vi "doStep.vi"(8 "error in (no error)":errorcluster, 10 "stepName":T1, 11 "Stand in":refnum<class "Stand.lvclass">) -> (0 "error out":errorcluster, 3 "Stand out":refnum<class "Stand.lvclass">)   [LabVIEW 2019, in "Stand.lvclass"]
uses:
  Stand.lvclass
  D:/GIT H4000/H4000/src/Device_class/Device.lvclass
  TypeDef/Step_Name.ctl
  Stand.lvclass/Stand.ctl
  Device_class/Device.lvclass/Device.ctl
  TypeDef/Direction.ctl
  FPGA/TypeDef/DO index.ctl
  FPGA/TypeDef/AI index.ctl
  AI_class/AI.lvclass/AI.ctl
  AnalogComparator_class/AnalogComparator.lvclass/AnalogComparator.ctl
  TypeDef/Active Motor.ctl
  TypeDef/Motor N.ctl
  f638fa31-f737-482a-bde8-81f5a2056bae.vi
  AnalogComparator_class/GetStatus.vi
  NeedleValve_class/NeedleValve.lvclass
  FPGA_API_class/FPGA API.lvclass
  MessageInterface_class/MessageInterface.lvclass
  Valve_2DO_2DI_class/Valve_2DO_2DI.lvclass
  Device_class/Device.lvclass
  PM_Group_class/PM_Group.lvclass
  AI_class/AI.lvclass
  ExpFitter/ExpFitter.lvclass
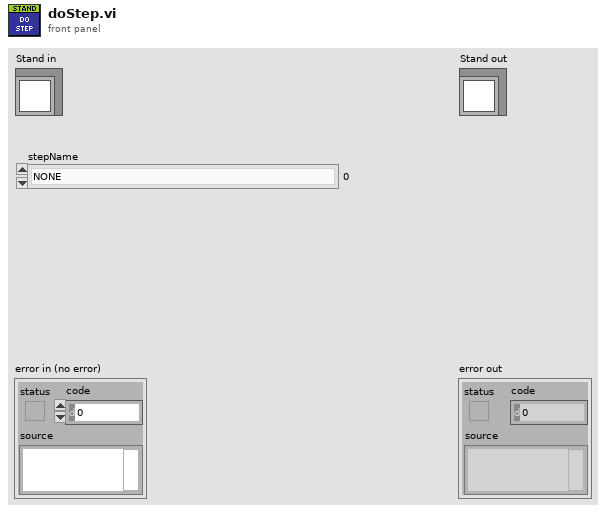
[diagram p1: front panel]
types:
  T1 = typedef "Step_Name.ctl" = enum16{"NONE", "Filling DUT", "Filling Chamber", "Pressure Up DUT", "Abrupt Pressure Release DUT", "Smooth Pressure Release DUT", "Pressure Up Chamber", "Abrupt Pressure Release Chamber", "Smooth Pressure Release Chamber", "Measuring leakage sensor 41.3", "Measuring leakage burette 42", "Low Pressure DUT", "Low Pressure Chamber", "Low Pressure HPP", "ALARM", "Open Air", "MicroStep DUT", "MicroStep CMBR", "Stop Pump"}
  T2 = typedef "Direction.ctl" = enum16{"None", "Chamber", "DUT"}
  T3 = typedef "Active Motor.ctl" = cluster{"Active":bool, "MotorN":T4}
  T4 = typedef "Motor N.ctl" = enum16{"M12", "M21", "M24"}
  T5 = typedef "DO index.ctl" = u8
  T6 = typedef "AI index.ctl" = u8
  T7 = typedef "AI_Data.ctl" = cluster{"Stat Data":T8, "OutOfRangeMax":bool, "OutOfRangeMin":bool, "HIHI":bool, "HI":bool, "LO":bool, "LOLO":bool}
  T8 = typedef "AI Statistics Data.ctl" = cluster{"raw mean":dbl, "scl mean":dbl, "raw mean 1Hz":dbl, "scl mean 1Hz":dbl, "raw standard deviation":dbl, "raw max value":dbl, "raw min value":dbl}
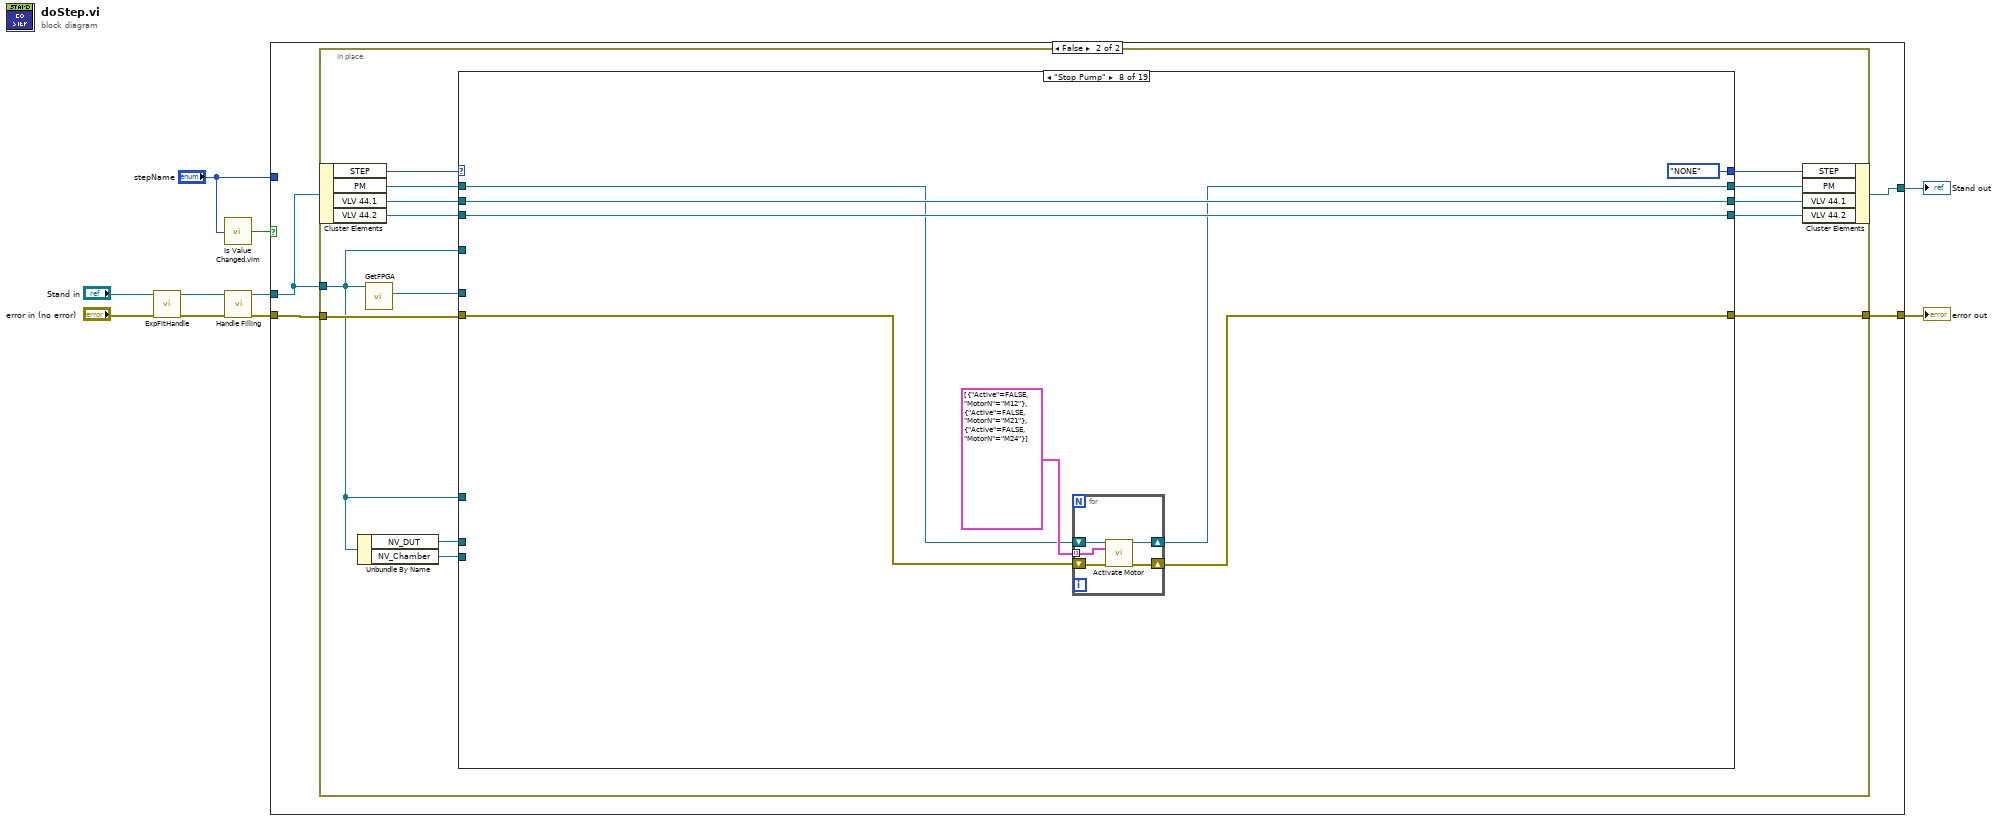
[diagram p0: block diagram]
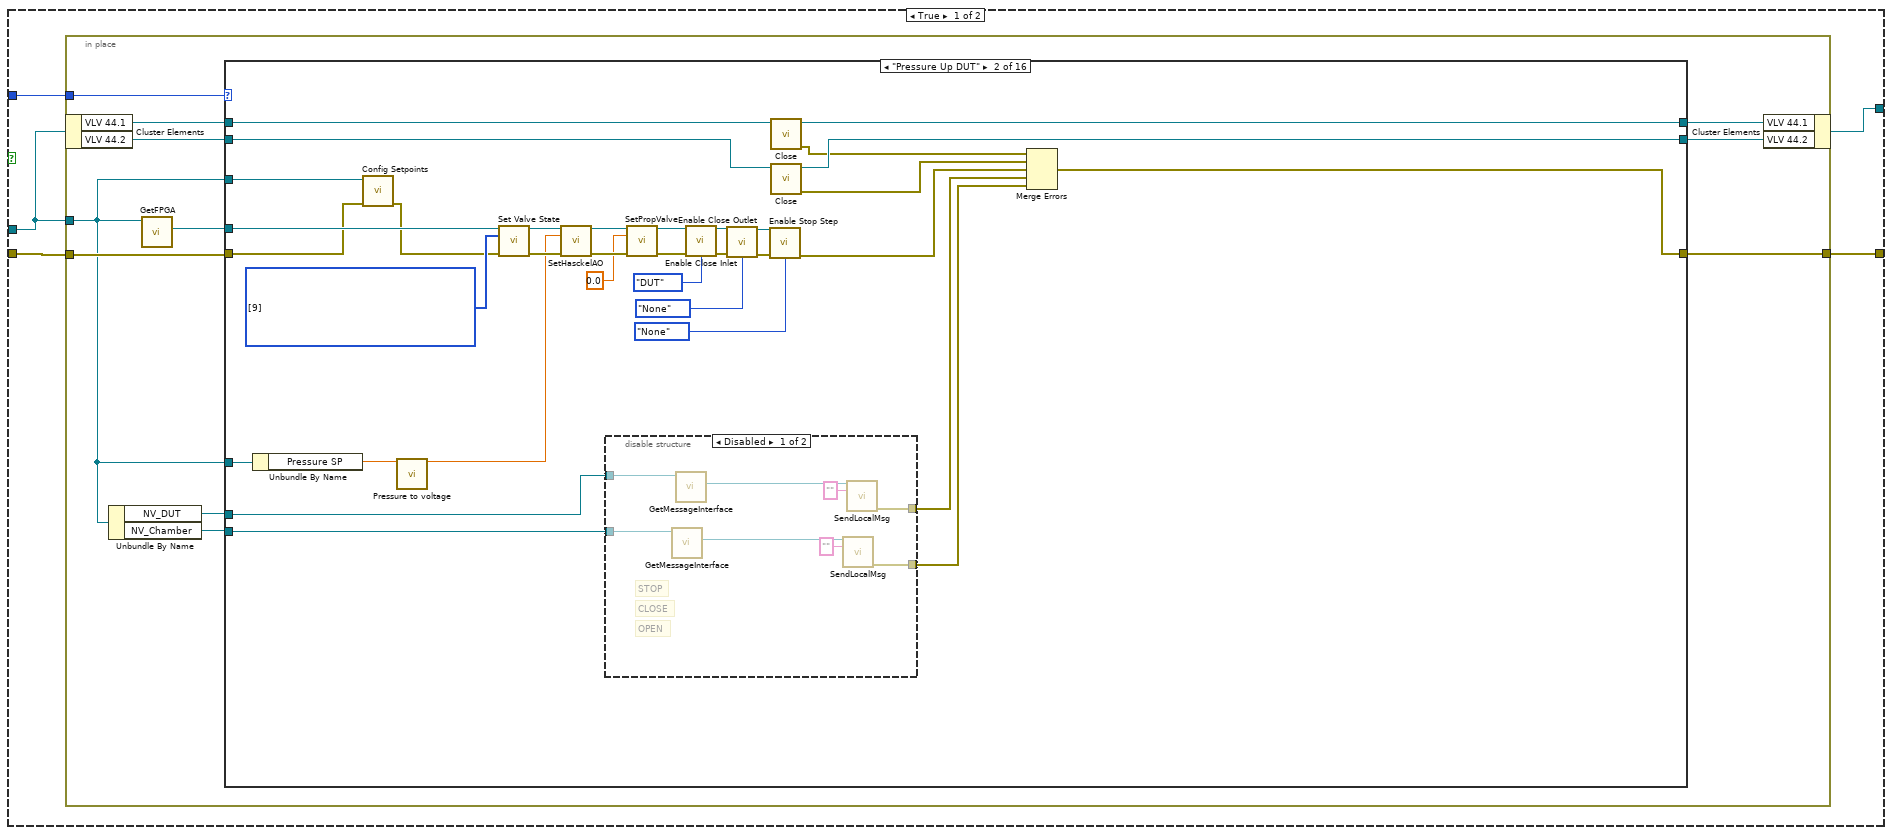
[diagram p2: hidden frame]
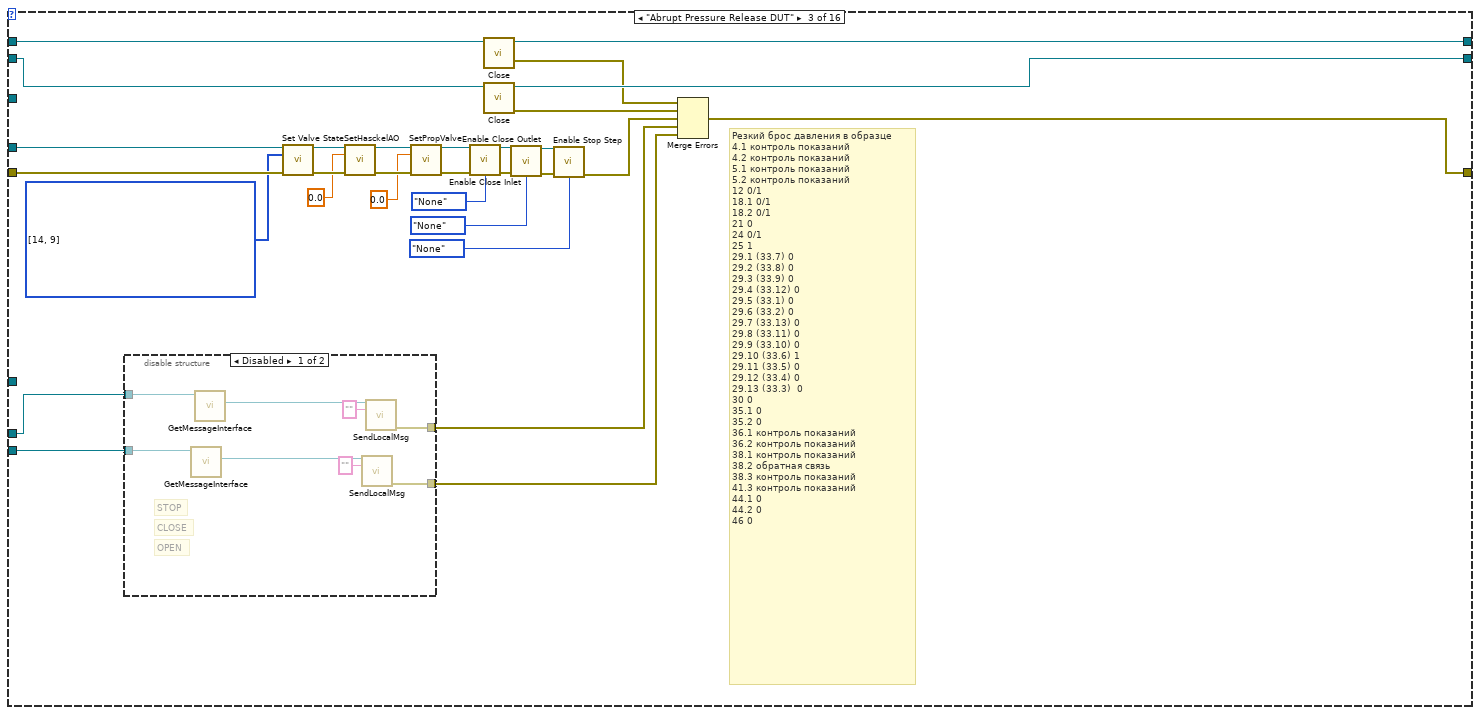
[diagram p5: hidden frame]
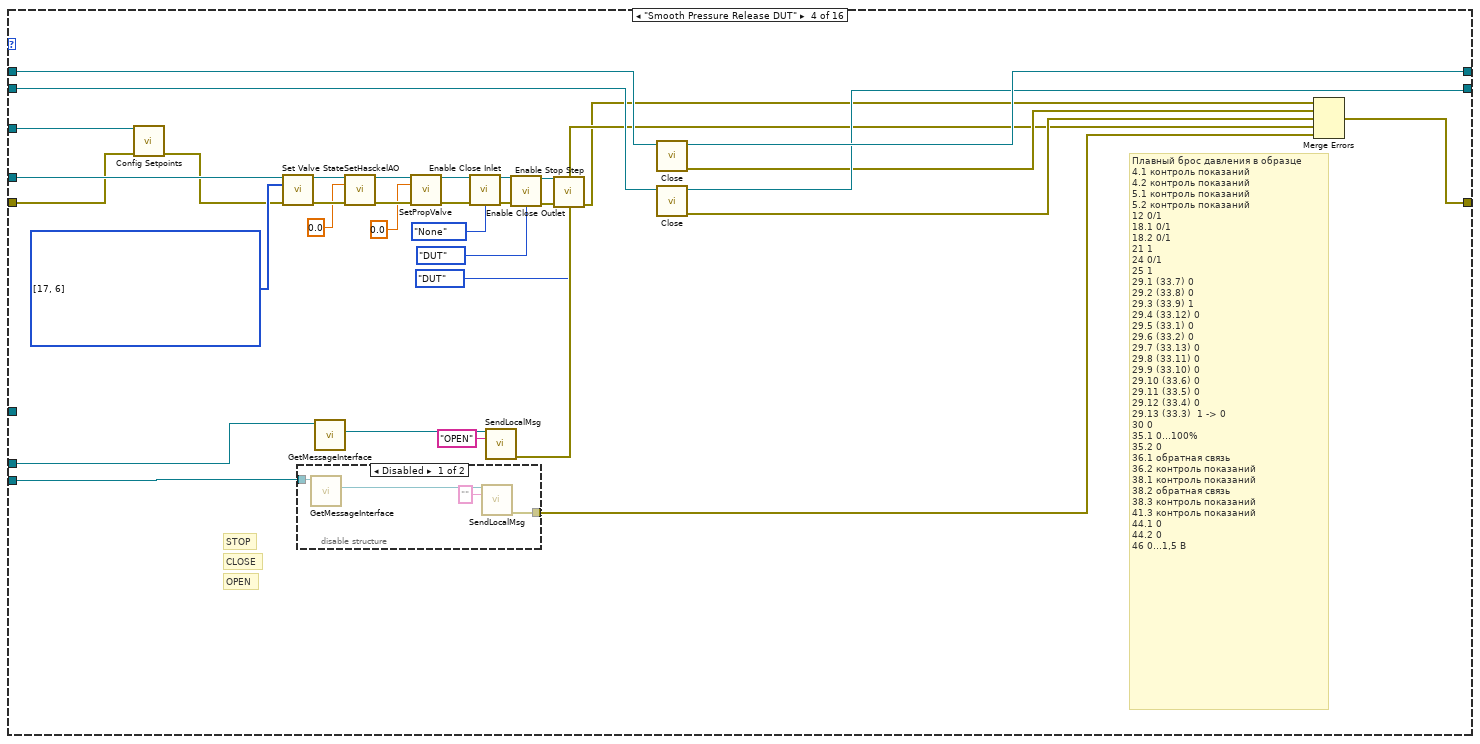
[diagram p7: hidden frame]
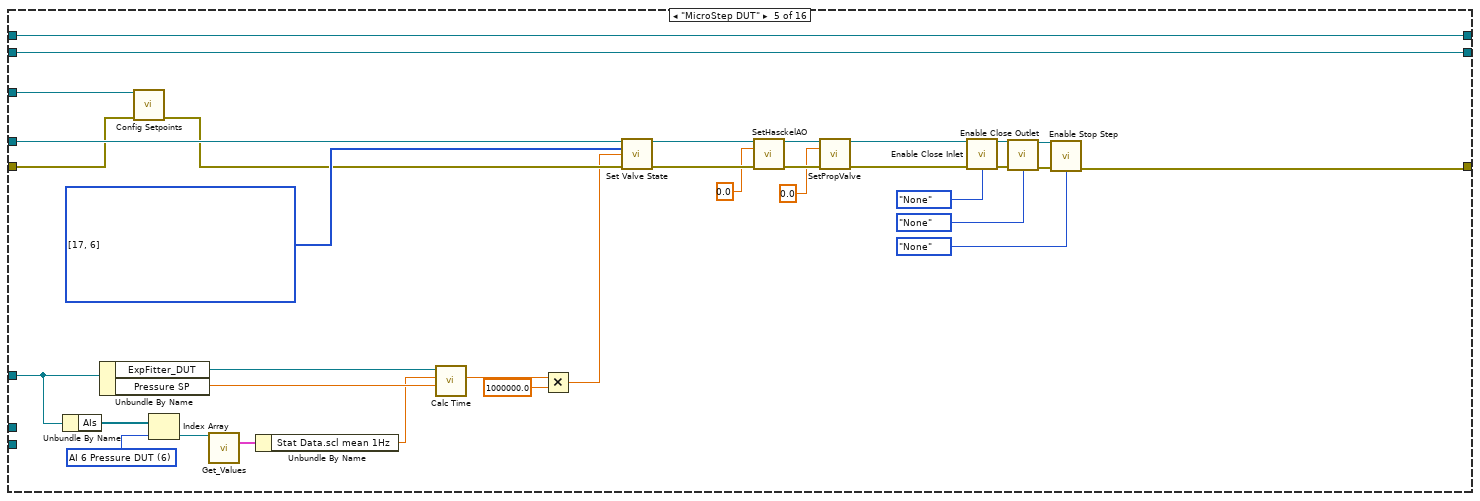
[diagram p9: hidden frame]
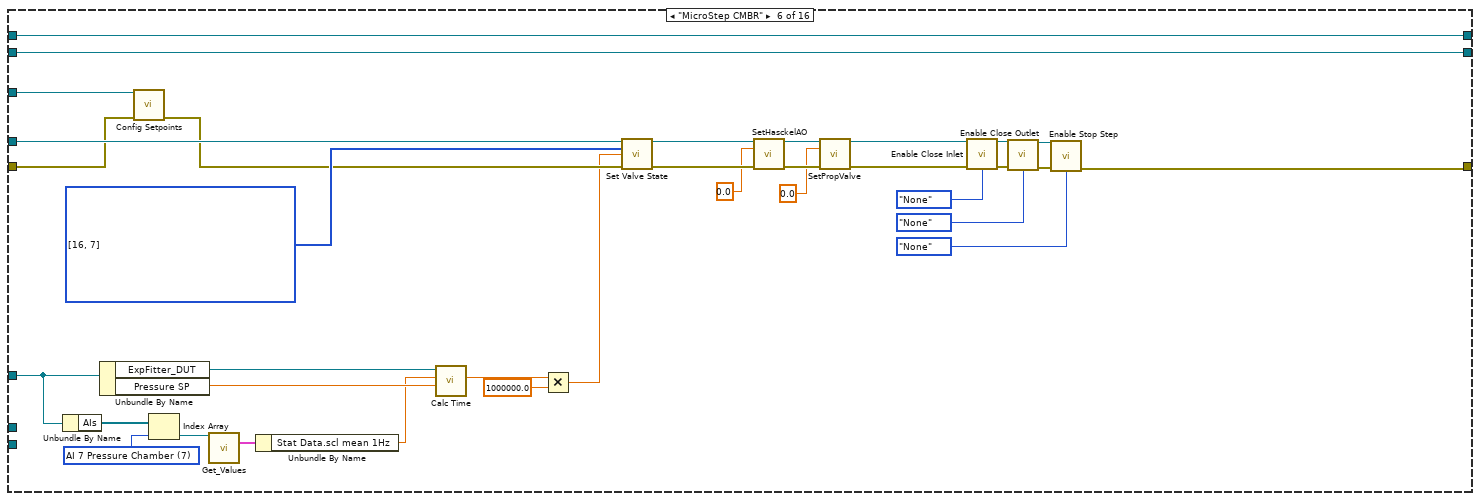
[diagram p10: hidden frame]
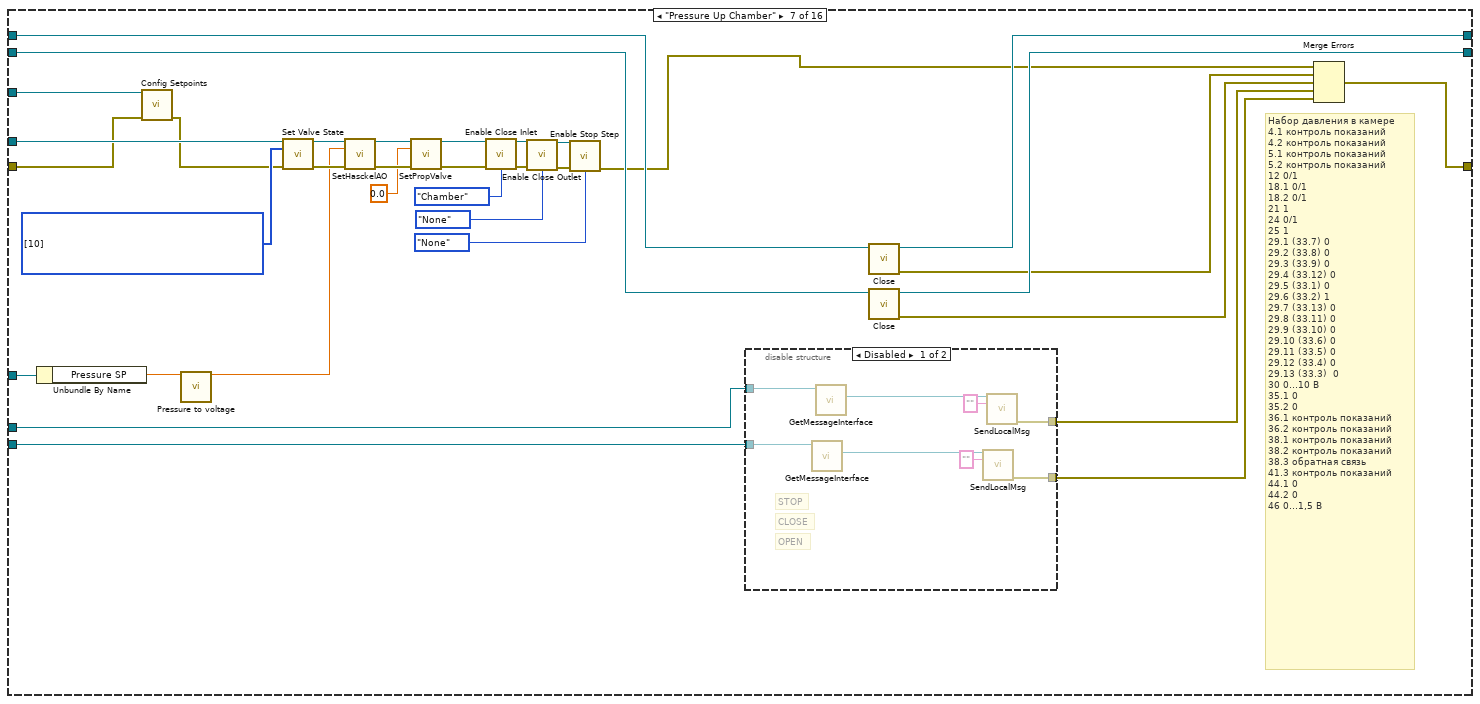
[diagram p11: hidden frame]
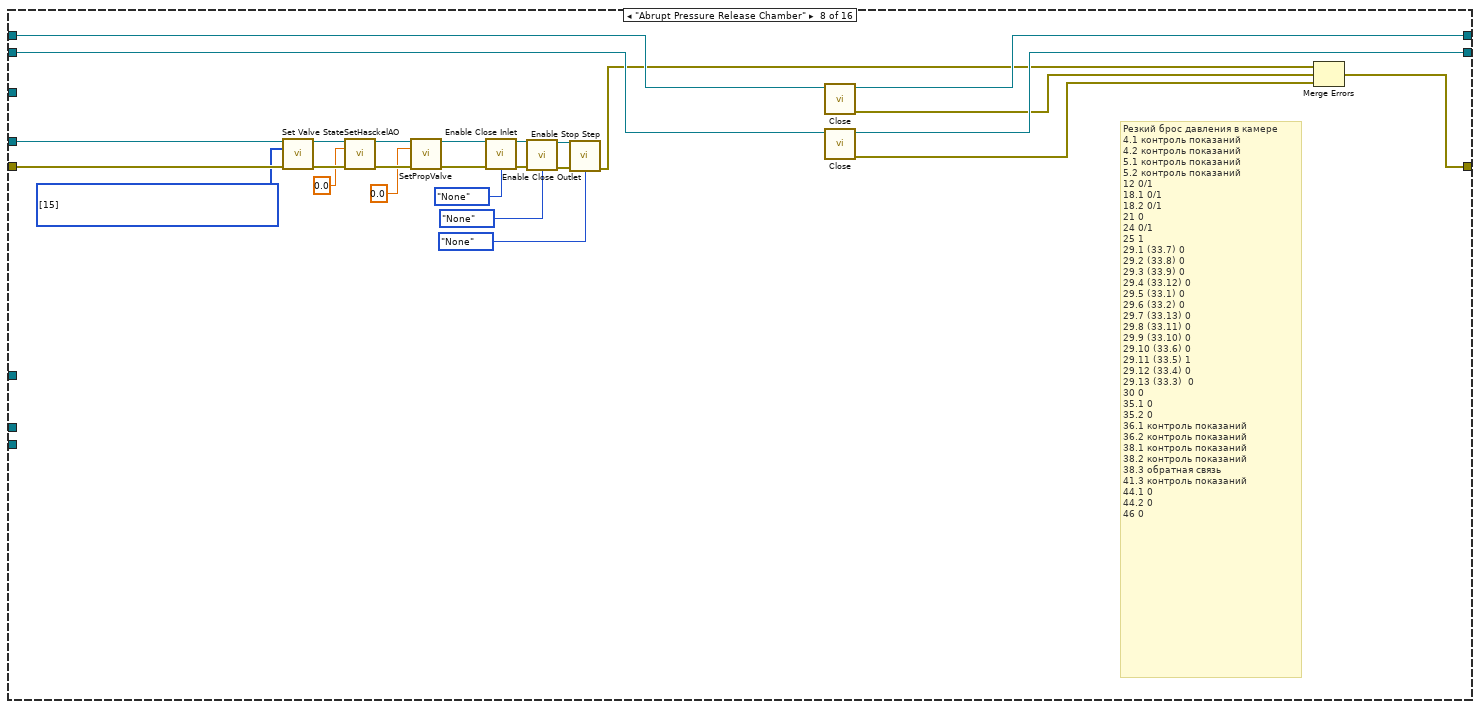
[diagram p13: hidden frame]
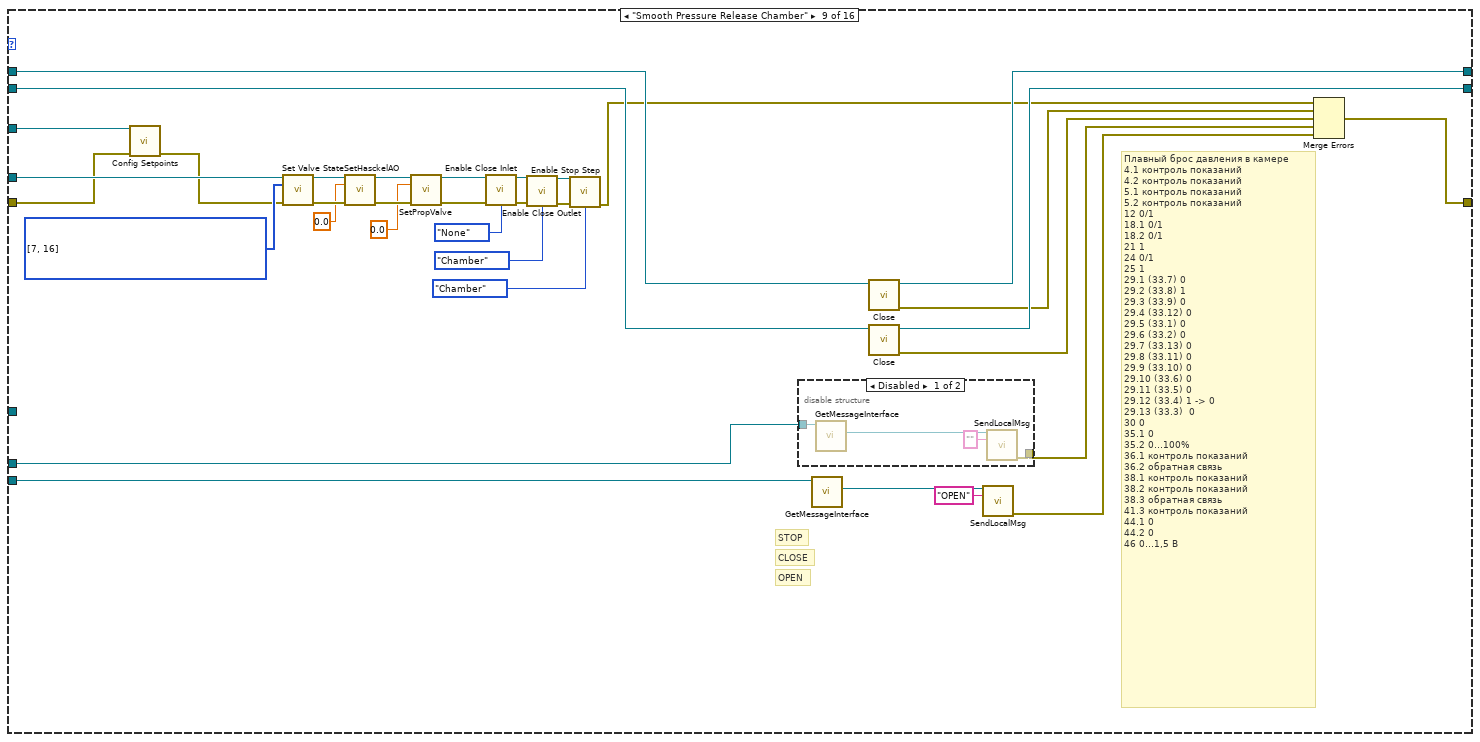
[diagram p14: hidden frame]
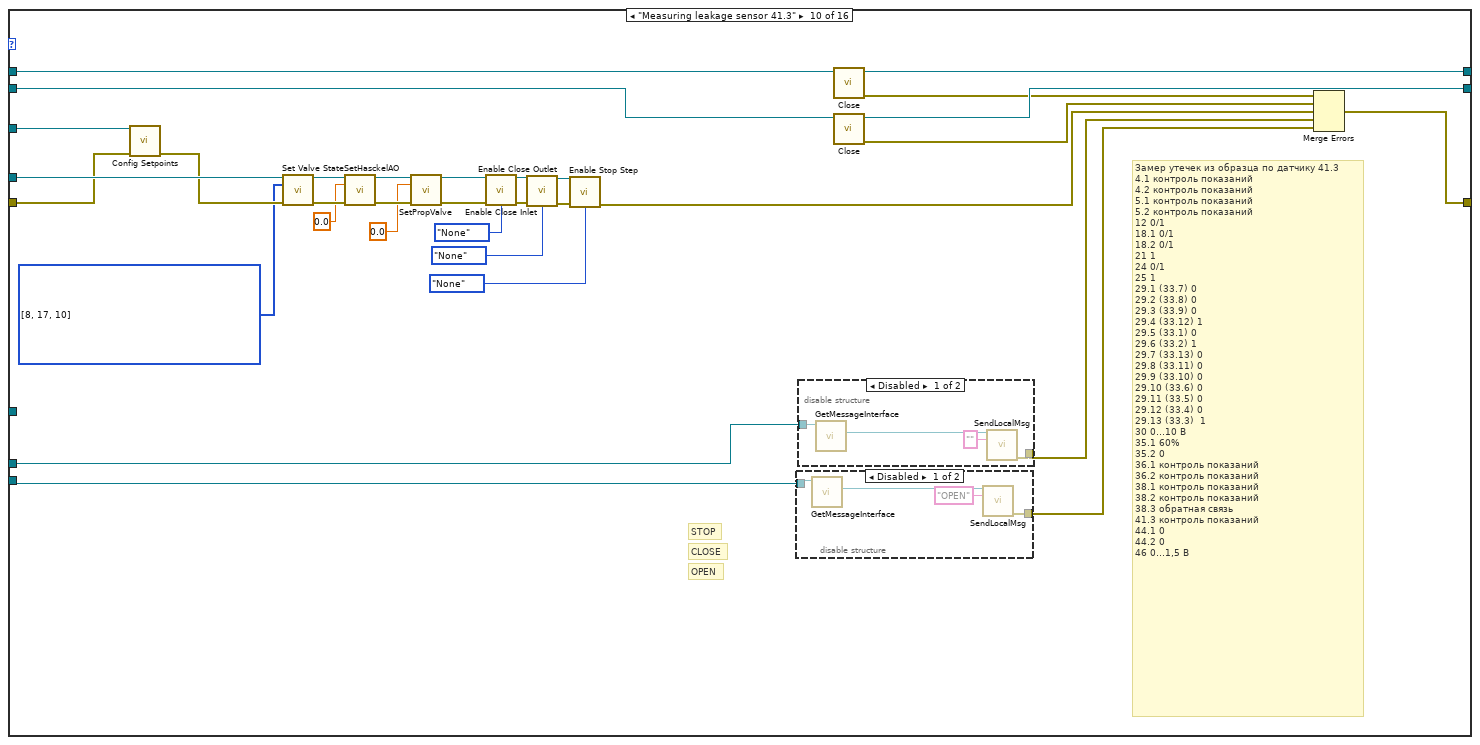
[diagram p16: hidden frame]
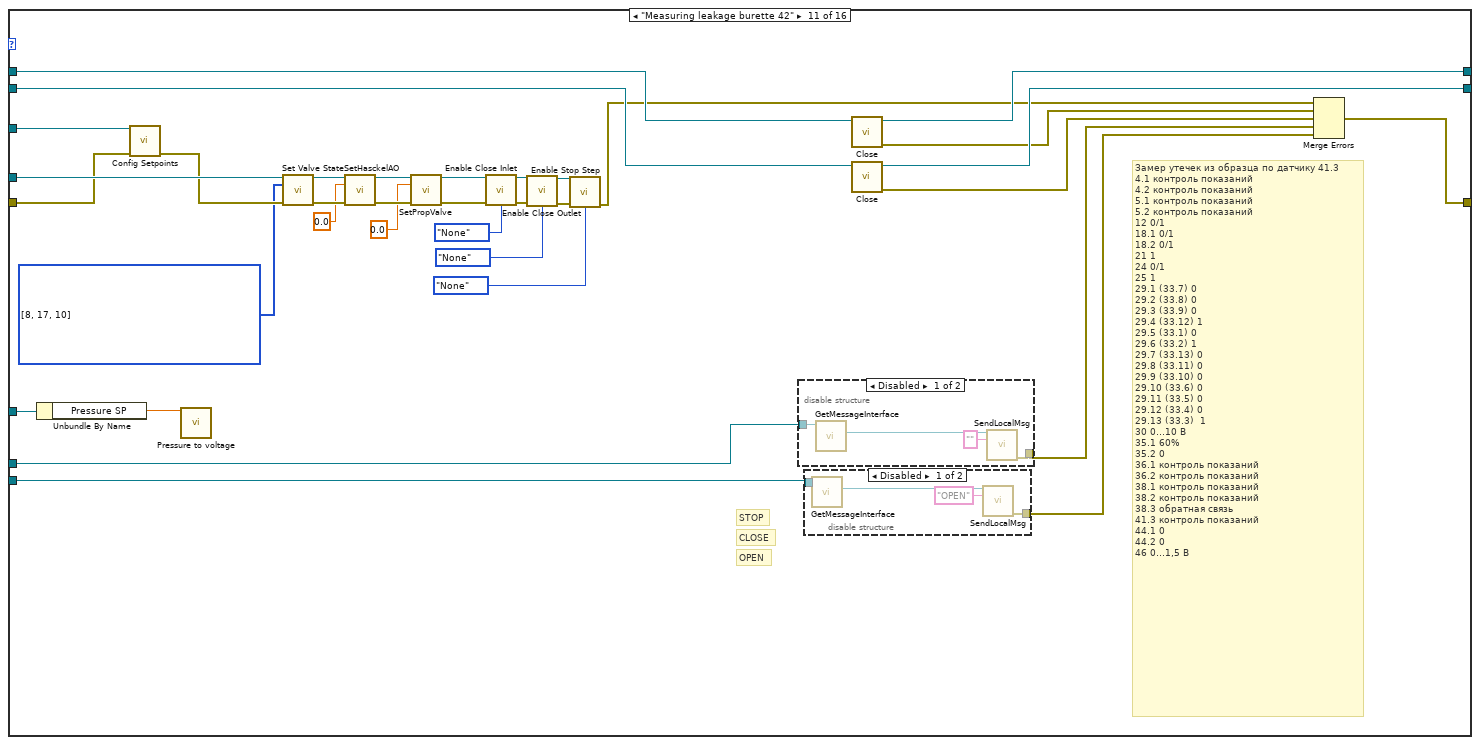
[diagram p19: hidden frame]
diagram:
  n1 = call "ExpFitHandle.vi"("error in (no error)"="error in (no error)", "Stand in"="Stand in") -> ("error out"=w3:errorcluster, "Stand out"=w4:refnum<class "Stand.lvclass">)  [unwired: 8 in]
  n2 = call "Is Value Changed.vim"("value"="stepName") -> ("changed or first call?"=w9:bool)
  n3 = call "Handle Filling.vi"("error in (no error)"=w3, "Stand in"=w4) -> ("error out"=w2:errorcluster, "Stand out"=w1:refnum<class "Stand.lvclass">)  [unwired: 8 in]
  n4 = case shown="False" w9 {
    tunnel: "stepName" -> [w15 _]
    tunnel: w1 -> [w13 w582]
    tunnel: w2 -> [w14 w583]
    tunnel: [w12 w581] -> w8
    tunnel: [w11 w580] -> w7
    frame True {
      n5 = in-place {
        in-place-border: w15 -> [w26]
        in-place-border: [w25] -> w11
        in-place-border: w14 -> [w24]
        in-place-border: w13 -> [w16]
        n6 = in-place-cluster #1(w13) -> ("VLV 44.1"=w22:refnum<class "Valve_2DO_2DI.lvclass">, "VLV 44.2"=w21:refnum<class "Valve_2DO_2DI.lvclass">)
        n7 = Unbundle By Name(w16) -> ("NV_DUT"=w18:refnum<class "NeedleValve.lvclass">, "NV_Chamber"=w17:refnum<class "NeedleValve.lvclass">)
        n8 = call "GetFPGA.vi"("Device in"=w16) -> ("FPGA API.lvclass"=w23:refnum<class "FPGA API.lvclass">)  [unwired: 10 in]
        n9 = case shown="\"Pressure Up DUT\"" w26 {
          tunnel: w24 -> [w29 w34 w101 w113 w160 w194 w217 w283 w285 w325 w364 w433 w471 w509 w543 w548]
          tunnel: [w29 w53 w91 w134 w166 w200 w239 w273 w308 w344 w385 w423 w461 w499 w533 w567] -> w25
          tunnel: w22 -> [w28 w58 w95 w138 w176 w210 w244 w277 w312 w348 w390 w427 w465 w503 w537 w569]
          tunnel: w21 -> [w27 w55 w93 w136 w175 w209 w241 w275 w310 w346 w387 w425 w463 w501 w535 w568]
          tunnel: w23 -> [_ w59 w96 w139 w177 w211 w245 w278 w313 w349 w391 w428 w466 w504 w538 w549]
          tunnel: w16 -> [_ w57 _ _ w153 w187 w243 _ _ _ w389 _ _ _ _ _]
          tunnel: [w28 w56 w94 w137 w176 w210 w242 w276 w311 w347 w388 w426 w464 w502 w536 w569] -> w20
          tunnel: [w27 w54 w92 w135 w175 w209 w240 w274 w309 w345 w386 w424 w462 w500 w534 w568] -> w19
          tunnel: w18 -> [_ w52 w90 w131 _ _ w236 _ w305 w341 w382 w420 w458 w496 _ w566]
          tunnel: w17 -> [_ w50 w88 w129 _ _ w234 _ w303 w339 w380 w418 w456 w494 _ w564]
          tunnel: w16 -> [_ w35 _ w114 w161 w195 w218 _ w286 w326 w365 _ _ _ _ _]
          frame "NONE", Default {
          }
          frame "Pressure Up DUT" {
            w39 = T5[] [9] items=["DO 0 [KP1] [M12]", "DO 1 [ON KP2] [M21]", "DO 2 [ON KP3] [M24]", "DO 3 [WATER Y18.1 [DO3]]", "DO 4 [WATER Y18.2 [DO4]]", "DO 5 [KP6 Y29.1 33.7]", "DO 6 [KP7 Y29.2 33.8]", "DO 7 [KP8 Y29.3 33.9]", "DO 8 [KP9 Y29.4  33.12]", "DO 9 [KP10 Y29.5 33.1]", "DO 10 [KP11 Y29.6 33.2]", "DO 11 [KP12 Y29.7  33.13]", "DO 12 [KP13 Y29.8  33.11]", "DO 13 [KP14 Y29.9 33.10]", "DO 14 [KP15 Y29.10  33.6]", "DO 15 [KP16 Y29.11  33.5]", "DO 16 [KP17 Y29.12  33.4]", "DO 17 [KP18 Y29.13 33.3]", "DO 18 [AIR KP19]", "DO 19 [STEP DRIVE EN KP20]", "DO 20 [KP21 Y44.1 OPEN]", "DO 21 [ KP22 Y44.1 CLOSE]", "DO 22 [ KP23 Y44.2 OPEN]", "DO 23", "DO 24 [STEP DRIVE 1]", "DO 25 [STEP DRIVE 2]"] ("#DO")
            n10 = Unbundle By Name(w57) -> ("Pressure SP"=w37:dbl)
            n11 = call "Config Setpoints.vi"("reference in"=w35, "error in (no error)"=w34) -> ("error out"=w33:errorcluster)  [unwired: 13 in]
            n12 = call "Pressure to voltage.vi"("Pressure SP"=w37) -> ("Voltage"=w36:dbl)  [unwired: 14 in]
            n13 = call "Set Valve State.vi"("reference in"=w59, "#DO"=w39, "error in (no error)"=w33) -> ("reference out"=w63:refnum<class "FPGA API.lvclass">, "error out"=w62:errorcluster)  [unwired: 11 in]
            n14 = call-dynamic "SetHasckelAO.vi"("FPGA API in"=w63, "Haskel in"=w36, "error in (no error)"=w62) -> ("FPGA API out"=w61:refnum<class "FPGA API.lvclass">, "error out"=w60:errorcluster)  [unwired: 11 in]
            n15 = disable-structure shown="Disabled" {
              disable-tunnel: w52 -> [w71 _]
              disable-tunnel: [w69 _] -> w51
              disable-tunnel: w50 -> [w67 _]
              disable-tunnel: [w64 _] -> w40
              frame Disabled {
                # "OPEN"
                # "CLOSE"
                # "STOP"
                n16 = call "GetMessageInterface.vi"("Device in"=w67) -> ("MessageInterface"=w68:refnum<class "MessageInterface.lvclass">)  [unwired: 10 in]
                n17 = call "GetMessageInterface.vi"("Device in"=w71) -> ("MessageInterface"=w70:refnum<class "MessageInterface.lvclass">)  [unwired: 10 in]
                n18 = call-dynamic "SendLocalMsg.vi"("reference in"=w68, "name"="") -> ("error out"=w64:errorcluster)  [unwired: 11 in, 2 out]
                n19 = call-dynamic "SendLocalMsg.vi"("reference in"=w70, "name"="") -> ("error out"=w69:errorcluster)  [unwired: 11 in, 2 out]
              }
              frame Enabled {
              }
            }
            n20 = call-dynamic "SetPropValve.vi"("FPGA API in"=w61, "AO 1"=0.0, "error in (no error)"=w60) -> ("FPGA API out"=w49:refnum<class "FPGA API.lvclass">, "error out"=w48:errorcluster)  [unwired: 11 in]
            n21 = call-dynamic "Enable Close Inlet.vi"("FPGA API in"=w49, "error in (no error)"=w48, "Direction"=Direction."DUT") -> ("FPGA API out"=w46:refnum<class "FPGA API.lvclass">, "error out"=w45:errorcluster)  [unwired: 11 in]
            n22 = call-dynamic "Enable Close Outlet.vi"("FPGA API in"=w46, "error in (no error)"=w45, "Direction"=Direction."None") -> ("FPGA API out"=w43:refnum<class "FPGA API.lvclass">, "error out"=w42:errorcluster)  [unwired: 11 in]
            n23 = call-dynamic "Enable Stop Step.vi"("FPGA API in"=w43, "error in (no error)"=w42, "Direction"=Direction."None") -> ("error out"=w32:errorcluster)  [unwired: 11 in, 1 out]
            n24 = call "Close.vi"("Pump_1AI_1DO_2DI in"=w58) -> ("error out"=w30:errorcluster, "Pump_1AI_1DO_2DI out"=w56:refnum<class "Valve_2DO_2DI.lvclass">)  [unwired: 9 in]
            n25 = call "Close.vi"("Pump_1AI_1DO_2DI in"=w55) -> ("error out"=w31:errorcluster, "Pump_1AI_1DO_2DI out"=w54:refnum<class "Valve_2DO_2DI.lvclass">)  [unwired: 9 in]
            n26 = Merge Errors(w30, w31, w32, w51, w40) -> (w53:errorcluster)
          }
          frame "Abrupt Pressure Release DUT" {
            w76 = T5[] [14, 9] items=["DO 0 [KP1] [M12]", "DO 1 [ON KP2] [M21]", "DO 2 [ON KP3] [M24]", "DO 3 [WATER Y18.1 [DO3]]", "DO 4 [WATER Y18.2 [DO4]]", "DO 5 [KP6 Y29.1 33.7]", "DO 6 [KP7 Y29.2 33.8]", "DO 7 [KP8 Y29.3 33.9]", "DO 8 [KP9 Y29.4  33.12]", "DO 9 [KP10 Y29.5 33.1]", "DO 10 [KP11 Y29.6 33.2]", "DO 11 [KP12 Y29.7  33.13]", "DO 12 [KP13 Y29.8  33.11]", "DO 13 [KP14 Y29.9 33.10]", "DO 14 [KP15 Y29.10  33.6]", "DO 15 [KP16 Y29.11  33.5]", "DO 16 [KP17 Y29.12  33.4]", "DO 17 [KP18 Y29.13 33.3]", "DO 18 [AIR KP19]", "DO 19 [STEP DRIVE EN KP20]", "DO 20 [KP21 Y44.1 OPEN]", "DO 21 [ KP22 Y44.1 CLOSE]", "DO 22 [ KP23 Y44.2 OPEN]", "DO 23", "DO 24 [STEP DRIVE 1]", "DO 25 [STEP DRIVE 2]"] ("#DO")
            # "Резкий брос давления в образце\n4.1\tконтроль показаний\n4.2\tконтроль показаний\n5.1\tконтроль показаний\n5.2\tконтроль показаний\n12\t0/1\n18.1\t0/1\n18.2\t0/1\n21\t0\n24\t0/1\n25\t1\n29.1 (33.7)\t0\n29.2 (33.8)\t0\n29.3 (33.9)\t0\n29.4 (33.12)\t0\n29.5 (33.1)\t0\n29.6 (33.2)\t0\n29.7 (33.13)\t0\n29.8 (33.11)\t0\n29.9 (33.10)\t0\n29.10 (33.6)\t1\n29.11 (33.5)\t0\n29.12 (33.4)\t0\n29.13 (33.3) \t0\n30\t0\n35.1\t0\n35.2\t0\n36.1\tконтроль показаний\n36.2\tконтроль показаний\n38.1\tконтроль показаний\n38.2\tобратная связь\n38.3\tконтроль показаний\n41.3\tконтроль показаний\n44.1\t0\n44.2\t0\n46\t0"
            n27 = disable-structure shown="Disabled" {
              disable-tunnel: w90 -> [w109 _]
              disable-tunnel: [w107 _] -> w89
              disable-tunnel: w88 -> [w105 _]
              disable-tunnel: [w102 _] -> w78
              frame Disabled {
                # "OPEN"
                # "CLOSE"
                # "STOP"
                n28 = call "GetMessageInterface.vi"("Device in"=w105) -> ("MessageInterface"=w106:refnum<class "MessageInterface.lvclass">)  [unwired: 10 in]
                n29 = call "GetMessageInterface.vi"("Device in"=w109) -> ("MessageInterface"=w108:refnum<class "MessageInterface.lvclass">)  [unwired: 10 in]
                n30 = call-dynamic "SendLocalMsg.vi"("reference in"=w106, "name"="") -> ("error out"=w102:errorcluster)  [unwired: 11 in, 2 out]
                n31 = call-dynamic "SendLocalMsg.vi"("reference in"=w108, "name"="") -> ("error out"=w107:errorcluster)  [unwired: 11 in, 2 out]
              }
              frame Enabled {
              }
            }
            n32 = call "Set Valve State.vi"("reference in"=w96, "#DO"=w76, "error in (no error)"=w101) -> ("reference out"=w100:refnum<class "FPGA API.lvclass">, "error out"=w99:errorcluster)  [unwired: 11 in]
            n33 = call-dynamic "SetHasckelAO.vi"("FPGA API in"=w100, "Haskel in"=0.0, "error in (no error)"=w99) -> ("FPGA API out"=w98:refnum<class "FPGA API.lvclass">, "error out"=w97:errorcluster)  [unwired: 11 in]
            n34 = call-dynamic "SetPropValve.vi"("FPGA API in"=w98, "AO 1"=0.0, "error in (no error)"=w97) -> ("FPGA API out"=w87:refnum<class "FPGA API.lvclass">, "error out"=w86:errorcluster)  [unwired: 11 in]
            n35 = call-dynamic "Enable Close Inlet.vi"("FPGA API in"=w87, "error in (no error)"=w86, "Direction"=Direction."None") -> ("FPGA API out"=w84:refnum<class "FPGA API.lvclass">, "error out"=w83:errorcluster)  [unwired: 11 in]
            n36 = call "Close.vi"("Pump_1AI_1DO_2DI in"=w95) -> ("error out"=w73:errorcluster, "Pump_1AI_1DO_2DI out"=w94:refnum<class "Valve_2DO_2DI.lvclass">)  [unwired: 9 in]
            n37 = call "Close.vi"("Pump_1AI_1DO_2DI in"=w93) -> ("error out"=w74:errorcluster, "Pump_1AI_1DO_2DI out"=w92:refnum<class "Valve_2DO_2DI.lvclass">)  [unwired: 9 in]
            n38 = call-dynamic "Enable Close Outlet.vi"("FPGA API in"=w84, "error in (no error)"=w83, "Direction"=Direction."None") -> ("FPGA API out"=w81:refnum<class "FPGA API.lvclass">, "error out"=w80:errorcluster)  [unwired: 11 in]
            n39 = call-dynamic "Enable Stop Step.vi"("FPGA API in"=w81, "error in (no error)"=w80, "Direction"=Direction."None") -> ("error out"=w72:errorcluster)  [unwired: 11 in, 1 out]
            n40 = Merge Errors(w73, w74, w72, w89, w78) -> (w91:errorcluster)
          }
          frame "Smooth Pressure Release DUT" {
            w116 = T5[] [17, 6] items=["DO 0 [KP1] [M12]", "DO 1 [ON KP2] [M21]", "DO 2 [ON KP3] [M24]", "DO 3 [WATER Y18.1 [DO3]]", "DO 4 [WATER Y18.2 [DO4]]", "DO 5 [KP6 Y29.1 33.7]", "DO 6 [KP7 Y29.2 33.8]", "DO 7 [KP8 Y29.3 33.9]", "DO 8 [KP9 Y29.4  33.12]", "DO 9 [KP10 Y29.5 33.1]", "DO 10 [KP11 Y29.6 33.2]", "DO 11 [KP12 Y29.7  33.13]", "DO 12 [KP13 Y29.8  33.11]", "DO 13 [KP14 Y29.9 33.10]", "DO 14 [KP15 Y29.10  33.6]", "DO 15 [KP16 Y29.11  33.5]", "DO 16 [KP17 Y29.12  33.4]", "DO 17 [KP18 Y29.13 33.3]", "DO 18 [AIR KP19]", "DO 19 [STEP DRIVE EN KP20]", "DO 20 [KP21 Y44.1 OPEN]", "DO 21 [ KP22 Y44.1 CLOSE]", "DO 22 [ KP23 Y44.2 OPEN]", "DO 23", "DO 24 [STEP DRIVE 1]", "DO 25 [STEP DRIVE 2]"] ("#DO")
            # "OPEN"
            # "CLOSE"
            # "STOP"
            # "Плавный брос давления в образце\n4.1\tконтроль показаний\n4.2\tконтроль показаний\n5.1\tконтроль показаний\n5.2\tконтроль показаний\n12\t0/1\n18.1\t0/1\n18.2\t0/1\n21\t1\n24\t0/1\n25\t1\n29.1 (33.7)\t0\n29.2 (33.8)\t0\n29.3 (33.9)\t1\n29.4 (33.12)\t0\n29.5 (33.1)\t0\n29.6 (33.2)\t0\n29.7 (33.13)\t0\n29.8 (33.11)\t0\n29.9 (33.10)\t0\n29.10 (33.6)\t0\n29.11 (33.5)\t0\n29.12 (33.4)\t0\n29.13 (33.3) \t1 -> 0\n30\t0\n35.1\t0…100%\n35.2\t0\n36.1\tобратная связь\n36.2\tконтроль показаний\n38.1\tконтроль показаний\n38.2\tобратная связь\n38.3\tконтроль показаний\n41.3\tконтроль показаний\n44.1\t0\n44.2\t0\n46\t0…1,5 В"
            n41 = call "Config Setpoints.vi"("reference in"=w114, "error in (no error)"=w113) -> ("error out"=w112:errorcluster)  [unwired: 13 in]
            n42 = call "Set Valve State.vi"("reference in"=w139, "#DO"=w116, "error in (no error)"=w112) -> ("reference out"=w143:refnum<class "FPGA API.lvclass">, "error out"=w142:errorcluster)  [unwired: 11 in]
            n43 = disable-structure shown="Disabled" {
              disable-tunnel: w129 -> [w147 _]
              disable-tunnel: [w146 _] -> w118
              frame Disabled {
                n44 = call "GetMessageInterface.vi"("Device in"=w147) -> ("MessageInterface"=w145:refnum<class "MessageInterface.lvclass">)  [unwired: 10 in]
                n45 = call-dynamic "SendLocalMsg.vi"("reference in"=w145, "name"="") -> ("error out"=w146:errorcluster)  [unwired: 11 in, 2 out]
              }
              frame Enabled {
              }
            }
            n46 = call "GetMessageInterface.vi"("Device in"=w131) -> ("MessageInterface"=w111:refnum<class "MessageInterface.lvclass">)  [unwired: 10 in]
            n47 = call-dynamic "SetHasckelAO.vi"("FPGA API in"=w143, "Haskel in"=0.0, "error in (no error)"=w142) -> ("FPGA API out"=w141:refnum<class "FPGA API.lvclass">, "error out"=w140:errorcluster)  [unwired: 11 in]
            n48 = call-dynamic "SetPropValve.vi"("FPGA API in"=w141, "AO 1"=0.0, "error in (no error)"=w140) -> ("FPGA API out"=w128:refnum<class "FPGA API.lvclass">, "error out"=w127:errorcluster)  [unwired: 11 in]
            n49 = call-dynamic "Enable Close Inlet.vi"("FPGA API in"=w128, "error in (no error)"=w127, "Direction"=Direction."None") -> ("FPGA API out"=w125:refnum<class "FPGA API.lvclass">, "error out"=w124:errorcluster)  [unwired: 11 in]
            n50 = call-dynamic "SendLocalMsg.vi"("reference in"=w111, "name"="OPEN") -> ("error out"=w130:errorcluster)  [unwired: 11 in, 2 out]
            n51 = call-dynamic "Enable Close Outlet.vi"("FPGA API in"=w125, "error in (no error)"=w124, "Direction"=Direction."DUT") -> ("FPGA API out"=w122:refnum<class "FPGA API.lvclass">, "error out"=w121:errorcluster)  [unwired: 11 in]
            n52 = call-dynamic "Enable Stop Step.vi"("FPGA API in"=w122, "error in (no error)"=w121, "Direction"=Direction."DUT") -> ("error out"=w120:errorcluster)  [unwired: 11 in, 1 out]
            n53 = call "Close.vi"("Pump_1AI_1DO_2DI in"=w138) -> ("error out"=w132:errorcluster, "Pump_1AI_1DO_2DI out"=w137:refnum<class "Valve_2DO_2DI.lvclass">)  [unwired: 9 in]
            n54 = call "Close.vi"("Pump_1AI_1DO_2DI in"=w136) -> ("error out"=w133:errorcluster, "Pump_1AI_1DO_2DI out"=w135:refnum<class "Valve_2DO_2DI.lvclass">)  [unwired: 9 in]
            n55 = Merge Errors(w120, w132, w133, w130, w118) -> (w134:errorcluster)
          }
          frame "MicroStep DUT" {
            w155 = T6 6 items=["AI 0 Cooling Station Level", "AI 1 Cooling Station Temp", "AI 2 Oil Supply Level", "AI 3 Oil Supply Temp", "AI 4 ", "AI 5 Pressure Haskel", "AI 6 Pressure DUT", "AI 7 Pressure Chamber", "AI 8 Pressure Air inlet", "AI 9 Pressure Air outlet", "AI 10 Pressure Messure Line"] ("AI index")
            w163 = T5[] [17, 6] items=["DO 0 [KP1] [M12]", "DO 1 [ON KP2] [M21]", "DO 2 [ON KP3] [M24]", "DO 3 [WATER Y18.1 [DO3]]", "DO 4 [WATER Y18.2 [DO4]]", "DO 5 [KP6 Y29.1 33.7]", "DO 6 [KP7 Y29.2 33.8]", "DO 7 [KP8 Y29.3 33.9]", "DO 8 [KP9 Y29.4  33.12]", "DO 9 [KP10 Y29.5 33.1]", "DO 10 [KP11 Y29.6 33.2]", "DO 11 [KP12 Y29.7  33.13]", "DO 12 [KP13 Y29.8  33.11]", "DO 13 [KP14 Y29.9 33.10]", "DO 14 [KP15 Y29.10  33.6]", "DO 15 [KP16 Y29.11  33.5]", "DO 16 [KP17 Y29.12  33.4]", "DO 17 [KP18 Y29.13 33.3]", "DO 18 [AIR KP19]", "DO 19 [STEP DRIVE EN KP20]", "DO 20 [KP21 Y44.1 OPEN]", "DO 21 [ KP22 Y44.1 CLOSE]", "DO 22 [ KP23 Y44.2 OPEN]", "DO 23", "DO 24 [STEP DRIVE 1]", "DO 25 [STEP DRIVE 2]"] ("#DO")
            n56 = Unbundle By Name(w153) -> ("AIs"=w154:refnum<class "AI.lvclass">[])
            n57 = Unbundle By Name(w153) -> ("ExpFitter_DUT"=w158:refnum<class "ExpFitter.lvclass">, "Pressure SP"=w152:dbl)
            n58 = call "Config Setpoints.vi"("reference in"=w161, "error in (no error)"=w160) -> ("error out"=w159:errorcluster)  [unwired: 13 in]
            n59 = Index Array(array=w154, index=w155) -> (element=w156:refnum<class "AI.lvclass">)
            n60 = call "Get_Values.vi"("reference in"=w156) -> ("Data"=w157:T7)  [unwired: 14 in]
            n61 = Unbundle By Name(w157) -> ("Stat Data.scl mean 1Hz"=w151:dbl)
            n62 = call "Calc Time.vi"("SP"=w152, "PV"=w151, "ExpFitter in"=w158) -> ("dT"=w150:dbl)  [unwired: 6 in, 2 out]
            n63 = Multiply(x=w150, y=1000000.0) -> (x*y=w148:dbl)
            n64 = call "Set Valve State.vi"("reference in"=w177, "#DO"=w163, "Time uSec"=w148, "error in (no error)"=w159) -> ("reference out"=w181:refnum<class "FPGA API.lvclass">, "error out"=w180:errorcluster)  [unwired: 10 in]
            n65 = call-dynamic "SetHasckelAO.vi"("FPGA API in"=w181, "Haskel in"=0.0, "error in (no error)"=w180) -> ("FPGA API out"=w179:refnum<class "FPGA API.lvclass">, "error out"=w178:errorcluster)  [unwired: 11 in]
            n66 = call-dynamic "SetPropValve.vi"("FPGA API in"=w179, "AO 1"=0.0, "error in (no error)"=w178) -> ("FPGA API out"=w174:refnum<class "FPGA API.lvclass">, "error out"=w173:errorcluster)  [unwired: 11 in]
            n67 = call-dynamic "Enable Close Inlet.vi"("FPGA API in"=w174, "error in (no error)"=w173, "Direction"=Direction."None") -> ("FPGA API out"=w171:refnum<class "FPGA API.lvclass">, "error out"=w170:errorcluster)  [unwired: 11 in]
            n68 = call-dynamic "Enable Close Outlet.vi"("FPGA API in"=w171, "error in (no error)"=w170, "Direction"=Direction."None") -> ("FPGA API out"=w168:refnum<class "FPGA API.lvclass">, "error out"=w167:errorcluster)  [unwired: 11 in]
            n69 = call-dynamic "Enable Stop Step.vi"("FPGA API in"=w168, "error in (no error)"=w167, "Direction"=Direction."None") -> ("error out"=w166:errorcluster)  [unwired: 11 in, 1 out]
          }
          frame "MicroStep CMBR" {
            w189 = T6 7 items=["AI 0 Cooling Station Level", "AI 1 Cooling Station Temp", "AI 2 Oil Supply Level", "AI 3 Oil Supply Temp", "AI 4 ", "AI 5 Pressure Haskel", "AI 6 Pressure DUT", "AI 7 Pressure Chamber", "AI 8 Pressure Air inlet", "AI 9 Pressure Air outlet", "AI 10 Pressure Messure Line"] ("AI index")
            w197 = T5[] [16, 7] items=["DO 0 [KP1] [M12]", "DO 1 [ON KP2] [M21]", "DO 2 [ON KP3] [M24]", "DO 3 [WATER Y18.1 [DO3]]", "DO 4 [WATER Y18.2 [DO4]]", "DO 5 [KP6 Y29.1 33.7]", "DO 6 [KP7 Y29.2 33.8]", "DO 7 [KP8 Y29.3 33.9]", "DO 8 [KP9 Y29.4  33.12]", "DO 9 [KP10 Y29.5 33.1]", "DO 10 [KP11 Y29.6 33.2]", "DO 11 [KP12 Y29.7  33.13]", "DO 12 [KP13 Y29.8  33.11]", "DO 13 [KP14 Y29.9 33.10]", "DO 14 [KP15 Y29.10  33.6]", "DO 15 [KP16 Y29.11  33.5]", "DO 16 [KP17 Y29.12  33.4]", "DO 17 [KP18 Y29.13 33.3]", "DO 18 [AIR KP19]", "DO 19 [STEP DRIVE EN KP20]", "DO 20 [KP21 Y44.1 OPEN]", "DO 21 [ KP22 Y44.1 CLOSE]", "DO 22 [ KP23 Y44.2 OPEN]", "DO 23", "DO 24 [STEP DRIVE 1]", "DO 25 [STEP DRIVE 2]"] ("#DO")
            n70 = Unbundle By Name(w187) -> ("AIs"=w188:refnum<class "AI.lvclass">[])
            n71 = Unbundle By Name(w187) -> ("ExpFitter_DUT"=w192:refnum<class "ExpFitter.lvclass">, "Pressure SP"=w186:dbl)
            n72 = call "Config Setpoints.vi"("reference in"=w195, "error in (no error)"=w194) -> ("error out"=w193:errorcluster)  [unwired: 13 in]
            n73 = Index Array(array=w188, index=w189) -> (element=w190:refnum<class "AI.lvclass">)
            n74 = call "Get_Values.vi"("reference in"=w190) -> ("Data"=w191:T7)  [unwired: 14 in]
            n75 = Unbundle By Name(w191) -> ("Stat Data.scl mean 1Hz"=w185:dbl)
            n76 = call "Calc Time.vi"("SP"=w186, "PV"=w185, "ExpFitter in"=w192) -> ("dT"=w184:dbl)  [unwired: 6 in, 2 out]
            n77 = Multiply(x=w184, y=1000000.0) -> (x*y=w182:dbl)
            n78 = call "Set Valve State.vi"("reference in"=w211, "#DO"=w197, "Time uSec"=w182, "error in (no error)"=w193) -> ("reference out"=w215:refnum<class "FPGA API.lvclass">, "error out"=w214:errorcluster)  [unwired: 10 in]
            n79 = call-dynamic "SetHasckelAO.vi"("FPGA API in"=w215, "Haskel in"=0.0, "error in (no error)"=w214) -> ("FPGA API out"=w213:refnum<class "FPGA API.lvclass">, "error out"=w212:errorcluster)  [unwired: 11 in]
            n80 = call-dynamic "SetPropValve.vi"("FPGA API in"=w213, "AO 1"=0.0, "error in (no error)"=w212) -> ("FPGA API out"=w208:refnum<class "FPGA API.lvclass">, "error out"=w207:errorcluster)  [unwired: 11 in]
            n81 = call-dynamic "Enable Close Inlet.vi"("FPGA API in"=w208, "error in (no error)"=w207, "Direction"=Direction."None") -> ("FPGA API out"=w205:refnum<class "FPGA API.lvclass">, "error out"=w204:errorcluster)  [unwired: 11 in]
            n82 = call-dynamic "Enable Close Outlet.vi"("FPGA API in"=w205, "error in (no error)"=w204, "Direction"=Direction."None") -> ("FPGA API out"=w202:refnum<class "FPGA API.lvclass">, "error out"=w201:errorcluster)  [unwired: 11 in]
            n83 = call-dynamic "Enable Stop Step.vi"("FPGA API in"=w202, "error in (no error)"=w201, "Direction"=Direction."None") -> ("error out"=w200:errorcluster)  [unwired: 11 in, 1 out]
          }
          frame "Pressure Up Chamber" {
            w219 = T5[] [10] items=["DO 0 [KP1] [M12]", "DO 1 [ON KP2] [M21]", "DO 2 [ON KP3] [M24]", "DO 3 [WATER Y18.1 [DO3]]", "DO 4 [WATER Y18.2 [DO4]]", "DO 5 [KP6 Y29.1 33.7]", "DO 6 [KP7 Y29.2 33.8]", "DO 7 [KP8 Y29.3 33.9]", "DO 8 [KP9 Y29.4  33.12]", "DO 9 [KP10 Y29.5 33.1]", "DO 10 [KP11 Y29.6 33.2]", "DO 11 [KP12 Y29.7  33.13]", "DO 12 [KP13 Y29.8  33.11]", "DO 13 [KP14 Y29.9 33.10]", "DO 14 [KP15 Y29.10  33.6]", "DO 15 [KP16 Y29.11  33.5]", "DO 16 [KP17 Y29.12  33.4]", "DO 17 [KP18 Y29.13 33.3]", "DO 18 [AIR KP19]", "DO 19 [STEP DRIVE EN KP20]", "DO 20 [KP21 Y44.1 OPEN]", "DO 21 [ KP22 Y44.1 CLOSE]", "DO 22 [ KP23 Y44.2 OPEN]", "DO 23", "DO 24 [STEP DRIVE 1]", "DO 25 [STEP DRIVE 2]"] ("#DO")
            # "Набор давления в камере\n4.1\tконтроль показаний\n4.2\tконтроль показаний\n5.1\tконтроль показаний\n5.2\tконтроль показаний\n12\t0/1\n18.1\t0/1\n18.2\t0/1\n21\t1\n24\t0/1\n25\t1\n29.1 (33.7)\t0\n29.2 (33.8)\t0\n29.3 (33.9)\t0\n29.4 (33.12)\t0\n29.5 (33.1)\t0\n29.6 (33.2)\t1\n29.7 (33.13)\t0\n29.8 (33.11)\t0\n29.9 (33.10)\t0\n29.10 (33.6)\t0\n29.11 (33.5)\t0\n29.12 (33.4)\t0\n29.13 (33.3) \t0\n30\t0…10 В\n35.1\t0\n35.2\t0\n36.1\tконтроль показаний\n36.2\tконтроль показаний\n38.1\tконтроль показаний\n38.2\tконтроль показаний\n38.3\tобратная связь\n41.3\tконтроль показаний\n44.1\t0\n44.2\t0\n46\t0…1,5 В"
            n84 = Unbundle By Name(w243) -> ("Pressure SP"=w221:dbl)
            n85 = call "Config Setpoints.vi"("reference in"=w218, "error in (no error)"=w217) -> ("error out"=w216:errorcluster)  [unwired: 13 in]
            n86 = call "Pressure to voltage.vi"("Pressure SP"=w221) -> ("Voltage"=w220:dbl)  [unwired: 14 in]
            n87 = call "Set Valve State.vi"("reference in"=w245, "#DO"=w219, "error in (no error)"=w216) -> ("reference out"=w249:refnum<class "FPGA API.lvclass">, "error out"=w248:errorcluster)  [unwired: 11 in]
            n88 = call-dynamic "SetHasckelAO.vi"("FPGA API in"=w249, "Haskel in"=w220, "error in (no error)"=w248) -> ("FPGA API out"=w247:refnum<class "FPGA API.lvclass">, "error out"=w246:errorcluster)  [unwired: 11 in]
            n89 = call-dynamic "SetPropValve.vi"("FPGA API in"=w247, "AO 1"=0.0, "error in (no error)"=w246) -> ("FPGA API out"=w233:refnum<class "FPGA API.lvclass">, "error out"=w232:errorcluster)  [unwired: 11 in]
            n90 = call-dynamic "Enable Close Inlet.vi"("FPGA API in"=w233, "error in (no error)"=w232, "Direction"=Direction."Chamber") -> ("FPGA API out"=w230:refnum<class "FPGA API.lvclass">, "error out"=w229:errorcluster)  [unwired: 11 in]
            n91 = call-dynamic "Enable Close Outlet.vi"("FPGA API in"=w230, "error in (no error)"=w229, "Direction"=Direction."None") -> ("FPGA API out"=w227:refnum<class "FPGA API.lvclass">, "error out"=w226:errorcluster)  [unwired: 11 in]
            n92 = call-dynamic "Enable Stop Step.vi"("FPGA API in"=w227, "error in (no error)"=w226, "Direction"=Direction."None") -> ("error out"=w225:errorcluster)  [unwired: 11 in, 1 out]
            n93 = disable-structure shown="Disabled" {
              disable-tunnel: w236 -> [w257 _]
              disable-tunnel: [w255 _] -> w235
              disable-tunnel: w234 -> [w253 _]
              disable-tunnel: [w250 _] -> w223
              frame Disabled {
                # "OPEN"
                # "CLOSE"
                # "STOP"
                n94 = call "GetMessageInterface.vi"("Device in"=w253) -> ("MessageInterface"=w254:refnum<class "MessageInterface.lvclass">)  [unwired: 10 in]
                n95 = call "GetMessageInterface.vi"("Device in"=w257) -> ("MessageInterface"=w256:refnum<class "MessageInterface.lvclass">)  [unwired: 10 in]
                n96 = call-dynamic "SendLocalMsg.vi"("reference in"=w254, "name"="") -> ("error out"=w250:errorcluster)  [unwired: 11 in, 2 out]
                n97 = call-dynamic "SendLocalMsg.vi"("reference in"=w256, "name"="") -> ("error out"=w255:errorcluster)  [unwired: 11 in, 2 out]
              }
              frame Enabled {
              }
            }
            n98 = call "Close.vi"("Pump_1AI_1DO_2DI in"=w244) -> ("error out"=w237:errorcluster, "Pump_1AI_1DO_2DI out"=w242:refnum<class "Valve_2DO_2DI.lvclass">)  [unwired: 9 in]
            n99 = call "Close.vi"("Pump_1AI_1DO_2DI in"=w241) -> ("error out"=w238:errorcluster, "Pump_1AI_1DO_2DI out"=w240:refnum<class "Valve_2DO_2DI.lvclass">)  [unwired: 9 in]
            n100 = Merge Errors(w225, w237, w238, w235, w223) -> (w239:errorcluster)
          }
          frame "Abrupt Pressure Release Chamber" {
            w259 = T5[] [15] items=["DO 0 [KP1] [M12]", "DO 1 [ON KP2] [M21]", "DO 2 [ON KP3] [M24]", "DO 3 [WATER Y18.1 [DO3]]", "DO 4 [WATER Y18.2 [DO4]]", "DO 5 [KP6 Y29.1 33.7]", "DO 6 [KP7 Y29.2 33.8]", "DO 7 [KP8 Y29.3 33.9]", "DO 8 [KP9 Y29.4  33.12]", "DO 9 [KP10 Y29.5 33.1]", "DO 10 [KP11 Y29.6 33.2]", "DO 11 [KP12 Y29.7  33.13]", "DO 12 [KP13 Y29.8  33.11]", "DO 13 [KP14 Y29.9 33.10]", "DO 14 [KP15 Y29.10  33.6]", "DO 15 [KP16 Y29.11  33.5]", "DO 16 [KP17 Y29.12  33.4]", "DO 17 [KP18 Y29.13 33.3]", "DO 18 [AIR KP19]", "DO 19 [STEP DRIVE EN KP20]", "DO 20 [KP21 Y44.1 OPEN]", "DO 21 [ KP22 Y44.1 CLOSE]", "DO 22 [ KP23 Y44.2 OPEN]", "DO 23", "DO 24 [STEP DRIVE 1]", "DO 25 [STEP DRIVE 2]"] ("#DO")
            # "Резкий брос давления в камере\n4.1\tконтроль показаний\n4.2\tконтроль показаний\n5.1\tконтроль показаний\n5.2\tконтроль показаний\n12\t0/1\n18.1\t0/1\n18.2\t0/1\n21\t0\n24\t0/1\n25\t1\n29.1 (33.7)\t0\n29.2 (33.8)\t0\n29.3 (33.9)\t0\n29.4 (33.12)\t0\n29.5 (33.1)\t0\n29.6 (33.2)\t0\n29.7 (33.13)\t0\n29.8 (33.11)\t0\n29.9 (33.10)\t0\n29.10 (33.6)\t0\n29.11 (33.5)\t1\n29.12 (33.4)\t0\n29.13 (33.3) \t0\n30\t0\n35.1\t0\n35.2\t0\n36.1\tконтроль показаний\n36.2\tконтроль показаний\n38.1\tконтроль показаний\n38.2\tконтроль показаний\n38.3\tобратная связь\n41.3\tконтроль показаний\n44.1\t0\n44.2\t0\n46\t0"
            n101 = call "Set Valve State.vi"("reference in"=w278, "#DO"=w259, "error in (no error)"=w283) -> ("reference out"=w282:refnum<class "FPGA API.lvclass">, "error out"=w281:errorcluster)  [unwired: 11 in]
            n102 = call-dynamic "SetHasckelAO.vi"("FPGA API in"=w282, "Haskel in"=0.0, "error in (no error)"=w281) -> ("FPGA API out"=w280:refnum<class "FPGA API.lvclass">, "error out"=w279:errorcluster)  [unwired: 11 in]
            n103 = call-dynamic "SetPropValve.vi"("FPGA API in"=w280, "AO 1"=0.0, "error in (no error)"=w279) -> ("FPGA API out"=w270:refnum<class "FPGA API.lvclass">, "error out"=w269:errorcluster)  [unwired: 11 in]
            n104 = call-dynamic "Enable Close Inlet.vi"("FPGA API in"=w270, "error in (no error)"=w269, "Direction"=Direction."None") -> ("FPGA API out"=w267:refnum<class "FPGA API.lvclass">, "error out"=w266:errorcluster)  [unwired: 11 in]
            n105 = call-dynamic "Enable Close Outlet.vi"("FPGA API in"=w267, "error in (no error)"=w266, "Direction"=Direction."None") -> ("FPGA API out"=w264:refnum<class "FPGA API.lvclass">, "error out"=w263:errorcluster)  [unwired: 11 in]
            n106 = call-dynamic "Enable Stop Step.vi"("FPGA API in"=w264, "error in (no error)"=w263, "Direction"=Direction."None") -> ("error out"=w262:errorcluster)  [unwired: 11 in, 1 out]
            n107 = call "Close.vi"("Pump_1AI_1DO_2DI in"=w277) -> ("error out"=w271:errorcluster, "Pump_1AI_1DO_2DI out"=w276:refnum<class "Valve_2DO_2DI.lvclass">)  [unwired: 9 in]
            n108 = call "Close.vi"("Pump_1AI_1DO_2DI in"=w275) -> ("error out"=w272:errorcluster, "Pump_1AI_1DO_2DI out"=w274:refnum<class "Valve_2DO_2DI.lvclass">)  [unwired: 9 in]
            n109 = Merge Errors(w262, w271, w272) -> (w273:errorcluster)
          }
          frame "Smooth Pressure Release Chamber" {
            w289 = T5[] [7, 16] items=["DO 0 [KP1] [M12]", "DO 1 [ON KP2] [M21]", "DO 2 [ON KP3] [M24]", "DO 3 [WATER Y18.1 [DO3]]", "DO 4 [WATER Y18.2 [DO4]]", "DO 5 [KP6 Y29.1 33.7]", "DO 6 [KP7 Y29.2 33.8]", "DO 7 [KP8 Y29.3 33.9]", "DO 8 [KP9 Y29.4  33.12]", "DO 9 [KP10 Y29.5 33.1]", "DO 10 [KP11 Y29.6 33.2]", "DO 11 [KP12 Y29.7  33.13]", "DO 12 [KP13 Y29.8  33.11]", "DO 13 [KP14 Y29.9 33.10]", "DO 14 [KP15 Y29.10  33.6]", "DO 15 [KP16 Y29.11  33.5]", "DO 16 [KP17 Y29.12  33.4]", "DO 17 [KP18 Y29.13 33.3]", "DO 18 [AIR KP19]", "DO 19 [STEP DRIVE EN KP20]", "DO 20 [KP21 Y44.1 OPEN]", "DO 21 [ KP22 Y44.1 CLOSE]", "DO 22 [ KP23 Y44.2 OPEN]", "DO 23", "DO 24 [STEP DRIVE 1]", "DO 25 [STEP DRIVE 2]"] ("#DO")
            # "OPEN"
            # "CLOSE"
            # "STOP"
            # "Плавный брос давления в камере\n4.1\tконтроль показаний\n4.2\tконтроль показаний\n5.1\tконтроль показаний\n5.2\tконтроль показаний\n12\t0/1\n18.1\t0/1\n18.2\t0/1\n21\t1\n24\t0/1\n25\t1\n29.1 (33.7)\t0\n29.2 (33.8)\t1\n29.3 (33.9)\t0\n29.4 (33.12)\t0\n29.5 (33.1)\t0\n29.6 (33.2)\t0\n29.7 (33.13)\t0\n29.8 (33.11)\t0\n29.9 (33.10)\t0\n29.10 (33.6)\t0\n29.11 (33.5)\t0\n29.12 (33.4)\t1 -> 0\n29.13 (33.3) \t0\n30\t0\n35.1\t0\n35.2\t0…100%\n36.1\tконтроль показаний\n36.2\tобратная связь\n38.1\tконтроль показаний\n38.2\tконтроль показаний\n38.3\tобратная связь\n41.3\tконтроль показаний\n44.1\t0\n44.2\t0\n46\t0…1,5 В"
            n110 = call "Config Setpoints.vi"("reference in"=w286, "error in (no error)"=w285) -> ("error out"=w284:errorcluster)  [unwired: 13 in]
            n111 = call "Set Valve State.vi"("reference in"=w313, "#DO"=w289, "error in (no error)"=w284) -> ("reference out"=w317:refnum<class "FPGA API.lvclass">, "error out"=w316:errorcluster)  [unwired: 11 in]
            n112 = call-dynamic "SetHasckelAO.vi"("FPGA API in"=w317, "Haskel in"=0.0, "error in (no error)"=w316) -> ("FPGA API out"=w315:refnum<class "FPGA API.lvclass">, "error out"=w314:errorcluster)  [unwired: 11 in]
            n113 = call-dynamic "SetPropValve.vi"("FPGA API in"=w315, "AO 1"=0.0, "error in (no error)"=w314) -> ("FPGA API out"=w302:refnum<class "FPGA API.lvclass">, "error out"=w301:errorcluster)  [unwired: 11 in]
            n114 = call-dynamic "Enable Close Inlet.vi"("FPGA API in"=w302, "error in (no error)"=w301, "Direction"=Direction."None") -> ("FPGA API out"=w299:refnum<class "FPGA API.lvclass">, "error out"=w298:errorcluster)  [unwired: 11 in]
            n115 = call-dynamic "Enable Close Outlet.vi"("FPGA API in"=w299, "error in (no error)"=w298, "Direction"=Direction."Chamber") -> ("FPGA API out"=w296:refnum<class "FPGA API.lvclass">, "error out"=w295:errorcluster)  [unwired: 11 in]
            n116 = call-dynamic "Enable Stop Step.vi"("FPGA API in"=w296, "error in (no error)"=w295, "Direction"=Direction."Chamber") -> ("error out"=w294:errorcluster)  [unwired: 11 in, 1 out]
            n117 = disable-structure shown="Disabled" {
              disable-tunnel: w305 -> [w321 _]
              disable-tunnel: [w320 _] -> w304
              frame Disabled {
                n118 = call "GetMessageInterface.vi"("Device in"=w321) -> ("MessageInterface"=w319:refnum<class "MessageInterface.lvclass">)  [unwired: 10 in]
                n119 = call-dynamic "SendLocalMsg.vi"("reference in"=w319, "name"="") -> ("error out"=w320:errorcluster)  [unwired: 11 in, 2 out]
              }
              frame Enabled {
              }
            }
            n120 = call "GetMessageInterface.vi"("Device in"=w303) -> ("MessageInterface"=w288:refnum<class "MessageInterface.lvclass">)  [unwired: 10 in]
            n121 = call "Close.vi"("Pump_1AI_1DO_2DI in"=w312) -> ("error out"=w306:errorcluster, "Pump_1AI_1DO_2DI out"=w311:refnum<class "Valve_2DO_2DI.lvclass">)  [unwired: 9 in]
            n122 = call "Close.vi"("Pump_1AI_1DO_2DI in"=w310) -> ("error out"=w307:errorcluster, "Pump_1AI_1DO_2DI out"=w309:refnum<class "Valve_2DO_2DI.lvclass">)  [unwired: 9 in]
            n123 = call-dynamic "SendLocalMsg.vi"("reference in"=w288, "name"="OPEN") -> ("error out"=w292:errorcluster)  [unwired: 11 in, 2 out]
            n124 = Merge Errors(w294, w306, w307, w304, w292) -> (w308:errorcluster)
          }
          frame "Measuring leakage sensor 41.3" {
            w323 = T5[] [8, 17, 10] items=["DO 0 [KP1] [M12]", "DO 1 [ON KP2] [M21]", "DO 2 [ON KP3] [M24]", "DO 3 [WATER Y18.1 [DO3]]", "DO 4 [WATER Y18.2 [DO4]]", "DO 5 [KP6 Y29.1 33.7]", "DO 6 [KP7 Y29.2 33.8]", "DO 7 [KP8 Y29.3 33.9]", "DO 8 [KP9 Y29.4  33.12]", "DO 9 [KP10 Y29.5 33.1]", "DO 10 [KP11 Y29.6 33.2]", "DO 11 [KP12 Y29.7  33.13]", "DO 12 [KP13 Y29.8  33.11]", "DO 13 [KP14 Y29.9 33.10]", "DO 14 [KP15 Y29.10  33.6]", "DO 15 [KP16 Y29.11  33.5]", "DO 16 [KP17 Y29.12  33.4]", "DO 17 [KP18 Y29.13 33.3]", "DO 18 [AIR KP19]", "DO 19 [STEP DRIVE EN KP20]", "DO 20 [KP21 Y44.1 OPEN]", "DO 21 [ KP22 Y44.1 CLOSE]", "DO 22 [ KP23 Y44.2 OPEN]", "DO 23", "DO 24 [STEP DRIVE 1]", "DO 25 [STEP DRIVE 2]"] ("#DO")
            # "Замер утечек из образца по датчику 41.3\n4.1\tконтроль показаний\n4.2\tконтроль показаний\n5.1\tконтроль показаний\n5.2\tконтроль показаний\n12\t0/1\n18.1\t0/1\n18.2\t0/1\n21\t1\n24\t0/1\n25\t1\n29.1 (33.7)\t0\n29.2 (33.8)\t0\n29.3 (33.9)\t0\n29.4 (33.12)\t1\n29.5 (33.1)\t0\n29.6 (33.2)\t1\n29.7 (33.13)\t0\n29.8 (33.11)\t0\n29.9 (33.10)\t0\n29.10 (33.6)\t0\n29.11 (33.5)\t0\n29.12 (33.4)\t0\n29.13 (33.3) \t1\n30\t0…10 В\n35.1\t60%\n35.2\t0\n36.1\tконтроль показаний\n36.2\tконтроль показаний\n38.1\tконтроль показаний\n38.2\tконтроль показаний\n38.3\tобратная связь\n41.3\tконтроль показаний\n44.1\t0\n44.2\t0\n46\t0…1,5 В"
            # "OPEN"
            # "CLOSE"
            # "STOP"
            n125 = call "Config Setpoints.vi"("reference in"=w326, "error in (no error)"=w325) -> ("error out"=w324:errorcluster)  [unwired: 13 in]
            n126 = call "Set Valve State.vi"("reference in"=w349, "#DO"=w323, "error in (no error)"=w324) -> ("reference out"=w353:refnum<class "FPGA API.lvclass">, "error out"=w352:errorcluster)  [unwired: 11 in]
            n127 = call-dynamic "SetHasckelAO.vi"("FPGA API in"=w353, "Haskel in"=0.0, "error in (no error)"=w352) -> ("FPGA API out"=w351:refnum<class "FPGA API.lvclass">, "error out"=w350:errorcluster)  [unwired: 11 in]
            n128 = call-dynamic "SetPropValve.vi"("FPGA API in"=w351, "AO 1"=0.0, "error in (no error)"=w350) -> ("FPGA API out"=w338:refnum<class "FPGA API.lvclass">, "error out"=w337:errorcluster)  [unwired: 11 in]
            n129 = call-dynamic "Enable Close Inlet.vi"("FPGA API in"=w338, "error in (no error)"=w337, "Direction"=Direction."None") -> ("FPGA API out"=w335:refnum<class "FPGA API.lvclass">, "error out"=w334:errorcluster)  [unwired: 11 in]
            n130 = call-dynamic "Enable Close Outlet.vi"("FPGA API in"=w335, "error in (no error)"=w334, "Direction"=Direction."None") -> ("FPGA API out"=w332:refnum<class "FPGA API.lvclass">, "error out"=w331:errorcluster)  [unwired: 11 in]
            n131 = call-dynamic "Enable Stop Step.vi"("FPGA API in"=w332, "error in (no error)"=w331, "Direction"=Direction."None") -> ("error out"=w322:errorcluster)  [unwired: 11 in, 1 out]
            n132 = disable-structure shown="Disabled" {
              disable-tunnel: w339 -> [w357 _]
              disable-tunnel: [w356 _] -> w329
              frame Disabled {
                n133 = call "GetMessageInterface.vi"("Device in"=w357) -> ("MessageInterface"=w355:refnum<class "MessageInterface.lvclass">)  [unwired: 10 in]
                n134 = call-dynamic "SendLocalMsg.vi"("reference in"=w355, "name"="OPEN") -> ("error out"=w356:errorcluster)  [unwired: 11 in, 2 out]
              }
              frame Enabled {
              }
            }
            n135 = disable-structure shown="Disabled" {
              disable-tunnel: w341 -> [w361 _]
              disable-tunnel: [w360 _] -> w340
              frame Disabled {
                n136 = call "GetMessageInterface.vi"("Device in"=w361) -> ("MessageInterface"=w359:refnum<class "MessageInterface.lvclass">)  [unwired: 10 in]
                n137 = call-dynamic "SendLocalMsg.vi"("reference in"=w359, "name"="") -> ("error out"=w360:errorcluster)  [unwired: 11 in, 2 out]
              }
              frame Enabled {
              }
            }
            n138 = call "Close.vi"("Pump_1AI_1DO_2DI in"=w348) -> ("error out"=w342:errorcluster, "Pump_1AI_1DO_2DI out"=w347:refnum<class "Valve_2DO_2DI.lvclass">)  [unwired: 9 in]
            n139 = call "Close.vi"("Pump_1AI_1DO_2DI in"=w346) -> ("error out"=w343:errorcluster, "Pump_1AI_1DO_2DI out"=w345:refnum<class "Valve_2DO_2DI.lvclass">)  [unwired: 9 in]
            n140 = Merge Errors(w342, w343, w322, w340, w329) -> (w344:errorcluster)
          }
          frame "Measuring leakage burette 42" {
            w362 = T5[] [8, 17, 10] items=["DO 0 [KP1] [M12]", "DO 1 [ON KP2] [M21]", "DO 2 [ON KP3] [M24]", "DO 3 [WATER Y18.1 [DO3]]", "DO 4 [WATER Y18.2 [DO4]]", "DO 5 [KP6 Y29.1 33.7]", "DO 6 [KP7 Y29.2 33.8]", "DO 7 [KP8 Y29.3 33.9]", "DO 8 [KP9 Y29.4  33.12]", "DO 9 [KP10 Y29.5 33.1]", "DO 10 [KP11 Y29.6 33.2]", "DO 11 [KP12 Y29.7  33.13]", "DO 12 [KP13 Y29.8  33.11]", "DO 13 [KP14 Y29.9 33.10]", "DO 14 [KP15 Y29.10  33.6]", "DO 15 [KP16 Y29.11  33.5]", "DO 16 [KP17 Y29.12  33.4]", "DO 17 [KP18 Y29.13 33.3]", "DO 18 [AIR KP19]", "DO 19 [STEP DRIVE EN KP20]", "DO 20 [KP21 Y44.1 OPEN]", "DO 21 [ KP22 Y44.1 CLOSE]", "DO 22 [ KP23 Y44.2 OPEN]", "DO 23", "DO 24 [STEP DRIVE 1]", "DO 25 [STEP DRIVE 2]"] ("#DO")
            # "Замер утечек из образца по датчику 41.3\n4.1\tконтроль показаний\n4.2\tконтроль показаний\n5.1\tконтроль показаний\n5.2\tконтроль показаний\n12\t0/1\n18.1\t0/1\n18.2\t0/1\n21\t1\n24\t0/1\n25\t1\n29.1 (33.7)\t0\n29.2 (33.8)\t0\n29.3 (33.9)\t0\n29.4 (33.12)\t1\n29.5 (33.1)\t0\n29.6 (33.2)\t1\n29.7 (33.13)\t0\n29.8 (33.11)\t0\n29.9 (33.10)\t0\n29.10 (33.6)\t0\n29.11 (33.5)\t0\n29.12 (33.4)\t0\n29.13 (33.3) \t1\n30\t0…10 В\n35.1\t60%\n35.2\t0\n36.1\tконтроль показаний\n36.2\tконтроль показаний\n38.1\tконтроль показаний\n38.2\tконтроль показаний\n38.3\tобратная связь\n41.3\tконтроль показаний\n44.1\t0\n44.2\t0\n46\t0…1,5 В"
            # "OPEN"
            # "CLOSE"
            # "STOP"
            n141 = Unbundle By Name(w389) -> ("Pressure SP"=w367:dbl)
            n142 = call "Config Setpoints.vi"("reference in"=w365, "error in (no error)"=w364) -> ("error out"=w363:errorcluster)  [unwired: 13 in]
            n143 = call "Pressure to voltage.vi"("Pressure SP"=w367) -> ()  [unwired: 14 in, 1 out]
            n144 = call "Set Valve State.vi"("reference in"=w391, "#DO"=w362, "error in (no error)"=w363) -> ("reference out"=w395:refnum<class "FPGA API.lvclass">, "error out"=w394:errorcluster)  [unwired: 11 in]
            n145 = call-dynamic "SetHasckelAO.vi"("FPGA API in"=w395, "Haskel in"=0.0, "error in (no error)"=w394) -> ("FPGA API out"=w393:refnum<class "FPGA API.lvclass">, "error out"=w392:errorcluster)  [unwired: 11 in]
            n146 = call-dynamic "SetPropValve.vi"("FPGA API in"=w393, "AO 1"=0.0, "error in (no error)"=w392) -> ("FPGA API out"=w379:refnum<class "FPGA API.lvclass">, "error out"=w378:errorcluster)  [unwired: 11 in]
            n147 = call-dynamic "Enable Close Inlet.vi"("FPGA API in"=w379, "error in (no error)"=w378, "Direction"=Direction."None") -> ("FPGA API out"=w376:refnum<class "FPGA API.lvclass">, "error out"=w375:errorcluster)  [unwired: 11 in]
            n148 = call-dynamic "Enable Close Outlet.vi"("FPGA API in"=w376, "error in (no error)"=w375, "Direction"=Direction."None") -> ("FPGA API out"=w373:refnum<class "FPGA API.lvclass">, "error out"=w372:errorcluster)  [unwired: 11 in]
            n149 = call-dynamic "Enable Stop Step.vi"("FPGA API in"=w373, "error in (no error)"=w372, "Direction"=Direction."None") -> ("error out"=w371:errorcluster)  [unwired: 11 in, 1 out]
            n150 = disable-structure shown="Disabled" {
              disable-tunnel: w382 -> [w403 _]
              disable-tunnel: [w402 _] -> w381
              frame Disabled {
                n151 = call "GetMessageInterface.vi"("Device in"=w403) -> ("MessageInterface"=w401:refnum<class "MessageInterface.lvclass">)  [unwired: 10 in]
                n152 = call-dynamic "SendLocalMsg.vi"("reference in"=w401, "name"="") -> ("error out"=w402:errorcluster)  [unwired: 11 in, 2 out]
              }
              frame Enabled {
              }
            }
            n153 = disable-structure shown="Disabled" {
              disable-tunnel: w380 -> [w399 _]
              disable-tunnel: [w398 _] -> w369
              frame Disabled {
                n154 = call "GetMessageInterface.vi"("Device in"=w399) -> ("MessageInterface"=w397:refnum<class "MessageInterface.lvclass">)  [unwired: 10 in]
                n155 = call-dynamic "SendLocalMsg.vi"("reference in"=w397, "name"="OPEN") -> ("error out"=w398:errorcluster)  [unwired: 11 in, 2 out]
              }
              frame Enabled {
              }
            }
            n156 = call "Close.vi"("Pump_1AI_1DO_2DI in"=w390) -> ("error out"=w383:errorcluster, "Pump_1AI_1DO_2DI out"=w388:refnum<class "Valve_2DO_2DI.lvclass">)  [unwired: 9 in]
            n157 = call "Close.vi"("Pump_1AI_1DO_2DI in"=w387) -> ("error out"=w384:errorcluster, "Pump_1AI_1DO_2DI out"=w386:refnum<class "Valve_2DO_2DI.lvclass">)  [unwired: 9 in]
            n158 = Merge Errors(w371, w383, w384, w381, w369) -> (w385:errorcluster)
          }
          frame "Low Pressure DUT" {
            w406 = T5[] [9, 5] items=["DO 0 [KP1] [M12]", "DO 1 [ON KP2] [M21]", "DO 2 [ON KP3] [M24]", "DO 3 [WATER Y18.1 [DO3]]", "DO 4 [WATER Y18.2 [DO4]]", "DO 5 [KP6 Y29.1 33.7]", "DO 6 [KP7 Y29.2 33.8]", "DO 7 [KP8 Y29.3 33.9]", "DO 8 [KP9 Y29.4  33.12]", "DO 9 [KP10 Y29.5 33.1]", "DO 10 [KP11 Y29.6 33.2]", "DO 11 [KP12 Y29.7  33.13]", "DO 12 [KP13 Y29.8  33.11]", "DO 13 [KP14 Y29.9 33.10]", "DO 14 [KP15 Y29.10  33.6]", "DO 15 [KP16 Y29.11  33.5]", "DO 16 [KP17 Y29.12  33.4]", "DO 17 [KP18 Y29.13 33.3]", "DO 18 [AIR KP19]", "DO 19 [STEP DRIVE EN KP20]", "DO 20 [KP21 Y44.1 OPEN]", "DO 21 [ KP22 Y44.1 CLOSE]", "DO 22 [ KP23 Y44.2 OPEN]", "DO 23", "DO 24 [STEP DRIVE 1]", "DO 25 [STEP DRIVE 2]"] ("#DO")
            n159 = call "Set Valve State.vi"("reference in"=w428, "#DO"=w406, "error in (no error)"=w433) -> ("reference out"=w432:refnum<class "FPGA API.lvclass">, "error out"=w431:errorcluster)  [unwired: 11 in]
            n160 = call-dynamic "SetHasckelAO.vi"("FPGA API in"=w432, "Haskel in"=0.0, "error in (no error)"=w431) -> ("FPGA API out"=w430:refnum<class "FPGA API.lvclass">, "error out"=w429:errorcluster)  [unwired: 11 in]
            n161 = call-dynamic "SetPropValve.vi"("FPGA API in"=w430, "AO 1"=0.0, "error in (no error)"=w429) -> ("FPGA API out"=w417:refnum<class "FPGA API.lvclass">, "error out"=w416:errorcluster)  [unwired: 11 in]
            n162 = call-dynamic "Enable Close Inlet.vi"("FPGA API in"=w417, "error in (no error)"=w416, "Direction"=Direction."None") -> ("FPGA API out"=w414:refnum<class "FPGA API.lvclass">, "error out"=w413:errorcluster)  [unwired: 11 in]
            n163 = call-dynamic "Enable Close Outlet.vi"("FPGA API in"=w414, "error in (no error)"=w413, "Direction"=Direction."None") -> ("FPGA API out"=w411:refnum<class "FPGA API.lvclass">, "error out"=w410:errorcluster)  [unwired: 11 in]
            n164 = call-dynamic "Enable Stop Step.vi"("FPGA API in"=w411, "error in (no error)"=w410, "Direction"=Direction."None") -> ("error out"=w409:errorcluster)  [unwired: 11 in, 1 out]
            n165 = disable-structure shown="Disabled" {
              disable-tunnel: w420 -> [w441 _]
              disable-tunnel: [w439 _] -> w419
              disable-tunnel: w418 -> [w437 _]
              disable-tunnel: [w434 _] -> w407
              frame Disabled {
                # "OPEN"
                # "CLOSE"
                # "STOP"
                n166 = call "GetMessageInterface.vi"("Device in"=w437) -> ("MessageInterface"=w438:refnum<class "MessageInterface.lvclass">)  [unwired: 10 in]
                n167 = call "GetMessageInterface.vi"("Device in"=w441) -> ("MessageInterface"=w440:refnum<class "MessageInterface.lvclass">)  [unwired: 10 in]
                n168 = call-dynamic "SendLocalMsg.vi"("reference in"=w438, "name"="") -> ("error out"=w434:errorcluster)  [unwired: 11 in, 2 out]
                n169 = call-dynamic "SendLocalMsg.vi"("reference in"=w440, "name"="") -> ("error out"=w439:errorcluster)  [unwired: 11 in, 2 out]
              }
              frame Enabled {
              }
            }
            n170 = call "Close.vi"("Pump_1AI_1DO_2DI in"=w427) -> ("error out"=w421:errorcluster, "Pump_1AI_1DO_2DI out"=w426:refnum<class "Valve_2DO_2DI.lvclass">)  [unwired: 9 in]
            n171 = call "Close.vi"("Pump_1AI_1DO_2DI in"=w425) -> ("error out"=w422:errorcluster, "Pump_1AI_1DO_2DI out"=w424:refnum<class "Valve_2DO_2DI.lvclass">)  [unwired: 9 in]
            n172 = Merge Errors(w409, w421, w422, w419, w407) -> (w423:errorcluster)
          }
          frame "Low Pressure Chamber" {
            w444 = T5[] [10, 5] items=["DO 0 [KP1] [M12]", "DO 1 [ON KP2] [M21]", "DO 2 [ON KP3] [M24]", "DO 3 [WATER Y18.1 [DO3]]", "DO 4 [WATER Y18.2 [DO4]]", "DO 5 [KP6 Y29.1 33.7]", "DO 6 [KP7 Y29.2 33.8]", "DO 7 [KP8 Y29.3 33.9]", "DO 8 [KP9 Y29.4  33.12]", "DO 9 [KP10 Y29.5 33.1]", "DO 10 [KP11 Y29.6 33.2]", "DO 11 [KP12 Y29.7  33.13]", "DO 12 [KP13 Y29.8  33.11]", "DO 13 [KP14 Y29.9 33.10]", "DO 14 [KP15 Y29.10  33.6]", "DO 15 [KP16 Y29.11  33.5]", "DO 16 [KP17 Y29.12  33.4]", "DO 17 [KP18 Y29.13 33.3]", "DO 18 [AIR KP19]", "DO 19 [STEP DRIVE EN KP20]", "DO 20 [KP21 Y44.1 OPEN]", "DO 21 [ KP22 Y44.1 CLOSE]", "DO 22 [ KP23 Y44.2 OPEN]", "DO 23", "DO 24 [STEP DRIVE 1]", "DO 25 [STEP DRIVE 2]"] ("#DO")
            n173 = call "Set Valve State.vi"("reference in"=w466, "#DO"=w444, "error in (no error)"=w471) -> ("reference out"=w470:refnum<class "FPGA API.lvclass">, "error out"=w469:errorcluster)  [unwired: 11 in]
            n174 = call-dynamic "SetHasckelAO.vi"("FPGA API in"=w470, "Haskel in"=0.0, "error in (no error)"=w469) -> ("FPGA API out"=w468:refnum<class "FPGA API.lvclass">, "error out"=w467:errorcluster)  [unwired: 11 in]
            n175 = call-dynamic "SetPropValve.vi"("FPGA API in"=w468, "AO 1"=0.0, "error in (no error)"=w467) -> ("FPGA API out"=w455:refnum<class "FPGA API.lvclass">, "error out"=w454:errorcluster)  [unwired: 11 in]
            n176 = call-dynamic "Enable Close Inlet.vi"("FPGA API in"=w455, "error in (no error)"=w454, "Direction"=Direction."None") -> ("FPGA API out"=w452:refnum<class "FPGA API.lvclass">, "error out"=w451:errorcluster)  [unwired: 11 in]
            n177 = call-dynamic "Enable Close Outlet.vi"("FPGA API in"=w452, "error in (no error)"=w451, "Direction"=Direction."None") -> ("FPGA API out"=w449:refnum<class "FPGA API.lvclass">, "error out"=w448:errorcluster)  [unwired: 11 in]
            n178 = call-dynamic "Enable Stop Step.vi"("FPGA API in"=w449, "error in (no error)"=w448, "Direction"=Direction."None") -> ("error out"=w447:errorcluster)  [unwired: 11 in, 1 out]
            n179 = disable-structure shown="Disabled" {
              disable-tunnel: w458 -> [w479 _]
              disable-tunnel: [w477 _] -> w457
              disable-tunnel: w456 -> [w475 _]
              disable-tunnel: [w472 _] -> w445
              frame Disabled {
                # "OPEN"
                # "CLOSE"
                # "STOP"
                n180 = call "GetMessageInterface.vi"("Device in"=w475) -> ("MessageInterface"=w476:refnum<class "MessageInterface.lvclass">)  [unwired: 10 in]
                n181 = call "GetMessageInterface.vi"("Device in"=w479) -> ("MessageInterface"=w478:refnum<class "MessageInterface.lvclass">)  [unwired: 10 in]
                n182 = call-dynamic "SendLocalMsg.vi"("reference in"=w476, "name"="") -> ("error out"=w472:errorcluster)  [unwired: 11 in, 2 out]
                n183 = call-dynamic "SendLocalMsg.vi"("reference in"=w478, "name"="") -> ("error out"=w477:errorcluster)  [unwired: 11 in, 2 out]
              }
              frame Enabled {
              }
            }
            n184 = call "Close.vi"("Pump_1AI_1DO_2DI in"=w465) -> ("error out"=w459:errorcluster, "Pump_1AI_1DO_2DI out"=w464:refnum<class "Valve_2DO_2DI.lvclass">)  [unwired: 9 in]
            n185 = call "Close.vi"("Pump_1AI_1DO_2DI in"=w463) -> ("error out"=w460:errorcluster, "Pump_1AI_1DO_2DI out"=w462:refnum<class "Valve_2DO_2DI.lvclass">)  [unwired: 9 in]
            n186 = Merge Errors(w447, w459, w460, w457, w445) -> (w461:errorcluster)
          }
          frame "Low Pressure HPP" {
            w482 = T5[] [5] items=["DO 0 [KP1] [M12]", "DO 1 [ON KP2] [M21]", "DO 2 [ON KP3] [M24]", "DO 3 [WATER Y18.1 [DO3]]", "DO 4 [WATER Y18.2 [DO4]]", "DO 5 [KP6 Y29.1 33.7]", "DO 6 [KP7 Y29.2 33.8]", "DO 7 [KP8 Y29.3 33.9]", "DO 8 [KP9 Y29.4  33.12]", "DO 9 [KP10 Y29.5 33.1]", "DO 10 [KP11 Y29.6 33.2]", "DO 11 [KP12 Y29.7  33.13]", "DO 12 [KP13 Y29.8  33.11]", "DO 13 [KP14 Y29.9 33.10]", "DO 14 [KP15 Y29.10  33.6]", "DO 15 [KP16 Y29.11  33.5]", "DO 16 [KP17 Y29.12  33.4]", "DO 17 [KP18 Y29.13 33.3]", "DO 18 [AIR KP19]", "DO 19 [STEP DRIVE EN KP20]", "DO 20 [KP21 Y44.1 OPEN]", "DO 21 [ KP22 Y44.1 CLOSE]", "DO 22 [ KP23 Y44.2 OPEN]", "DO 23", "DO 24 [STEP DRIVE 1]", "DO 25 [STEP DRIVE 2]"] ("#DO")
            n187 = call "Set Valve State.vi"("reference in"=w504, "#DO"=w482, "error in (no error)"=w509) -> ("reference out"=w508:refnum<class "FPGA API.lvclass">, "error out"=w507:errorcluster)  [unwired: 11 in]
            n188 = call-dynamic "SetHasckelAO.vi"("FPGA API in"=w508, "Haskel in"=0.0, "error in (no error)"=w507) -> ("FPGA API out"=w506:refnum<class "FPGA API.lvclass">, "error out"=w505:errorcluster)  [unwired: 11 in]
            n189 = call-dynamic "SetPropValve.vi"("FPGA API in"=w506, "AO 1"=0.0, "error in (no error)"=w505) -> ("FPGA API out"=w493:refnum<class "FPGA API.lvclass">, "error out"=w492:errorcluster)  [unwired: 11 in]
            n190 = call-dynamic "Enable Close Inlet.vi"("FPGA API in"=w493, "error in (no error)"=w492, "Direction"=Direction."None") -> ("FPGA API out"=w490:refnum<class "FPGA API.lvclass">, "error out"=w489:errorcluster)  [unwired: 11 in]
            n191 = call-dynamic "Enable Close Outlet.vi"("FPGA API in"=w490, "error in (no error)"=w489, "Direction"=Direction."None") -> ("FPGA API out"=w487:refnum<class "FPGA API.lvclass">, "error out"=w486:errorcluster)  [unwired: 11 in]
            n192 = call-dynamic "Enable Stop Step.vi"("FPGA API in"=w487, "error in (no error)"=w486, "Direction"=Direction."None") -> ("error out"=w485:errorcluster)  [unwired: 11 in, 1 out]
            n193 = disable-structure shown="Disabled" {
              disable-tunnel: w496 -> [w517 _]
              disable-tunnel: [w515 _] -> w495
              disable-tunnel: w494 -> [w513 _]
              disable-tunnel: [w510 _] -> w483
              frame Disabled {
                # "OPEN"
                # "CLOSE"
                # "STOP"
                n194 = call "GetMessageInterface.vi"("Device in"=w513) -> ("MessageInterface"=w514:refnum<class "MessageInterface.lvclass">)  [unwired: 10 in]
                n195 = call "GetMessageInterface.vi"("Device in"=w517) -> ("MessageInterface"=w516:refnum<class "MessageInterface.lvclass">)  [unwired: 10 in]
                n196 = call-dynamic "SendLocalMsg.vi"("reference in"=w514, "name"="") -> ("error out"=w510:errorcluster)  [unwired: 11 in, 2 out]
                n197 = call-dynamic "SendLocalMsg.vi"("reference in"=w516, "name"="") -> ("error out"=w515:errorcluster)  [unwired: 11 in, 2 out]
              }
              frame Enabled {
              }
            }
            n198 = call "Close.vi"("Pump_1AI_1DO_2DI in"=w503) -> ("error out"=w497:errorcluster, "Pump_1AI_1DO_2DI out"=w502:refnum<class "Valve_2DO_2DI.lvclass">)  [unwired: 9 in]
            n199 = call "Close.vi"("Pump_1AI_1DO_2DI in"=w501) -> ("error out"=w498:errorcluster, "Pump_1AI_1DO_2DI out"=w500:refnum<class "Valve_2DO_2DI.lvclass">)  [unwired: 9 in]
            n200 = Merge Errors(w485, w497, w498, w495, w483) -> (w499:errorcluster)
          }
          frame "ALARM" {
            w520 = T5[] [15, 14, 9, 10] items=["DO 0 [KP1] [M12]", "DO 1 [ON KP2] [M21]", "DO 2 [ON KP3] [M24]", "DO 3 [WATER Y18.1 [DO3]]", "DO 4 [WATER Y18.2 [DO4]]", "DO 5 [KP6 Y29.1 33.7]", "DO 6 [KP7 Y29.2 33.8]", "DO 7 [KP8 Y29.3 33.9]", "DO 8 [KP9 Y29.4  33.12]", "DO 9 [KP10 Y29.5 33.1]", "DO 10 [KP11 Y29.6 33.2]", "DO 11 [KP12 Y29.7  33.13]", "DO 12 [KP13 Y29.8  33.11]", "DO 13 [KP14 Y29.9 33.10]", "DO 14 [KP15 Y29.10  33.6]", "DO 15 [KP16 Y29.11  33.5]", "DO 16 [KP17 Y29.12  33.4]", "DO 17 [KP18 Y29.13 33.3]", "DO 18 [AIR KP19]", "DO 19 [STEP DRIVE EN KP20]", "DO 20 [KP21 Y44.1 OPEN]", "DO 21 [ KP22 Y44.1 CLOSE]", "DO 22 [ KP23 Y44.2 OPEN]", "DO 23", "DO 24 [STEP DRIVE 1]", "DO 25 [STEP DRIVE 2]"] ("#DO")
            n201 = call "Set Valve State.vi"("reference in"=w538, "#DO"=w520, "error in (no error)"=w543) -> ("reference out"=w542:refnum<class "FPGA API.lvclass">, "error out"=w541:errorcluster)  [unwired: 11 in]
            n202 = call-dynamic "SetHasckelAO.vi"("FPGA API in"=w542, "Haskel in"=0.0, "error in (no error)"=w541) -> ("FPGA API out"=w540:refnum<class "FPGA API.lvclass">, "error out"=w539:errorcluster)  [unwired: 11 in]
            n203 = call-dynamic "SetPropValve.vi"("FPGA API in"=w540, "AO 1"=0.0, "error in (no error)"=w539) -> ("FPGA API out"=w530:refnum<class "FPGA API.lvclass">, "error out"=w529:errorcluster)  [unwired: 11 in]
            n204 = call-dynamic "Enable Close Inlet.vi"("FPGA API in"=w530, "error in (no error)"=w529, "Direction"=Direction."None") -> ("FPGA API out"=w527:refnum<class "FPGA API.lvclass">, "error out"=w526:errorcluster)  [unwired: 11 in]
            n205 = call-dynamic "Enable Close Outlet.vi"("FPGA API in"=w527, "error in (no error)"=w526, "Direction"=Direction."None") -> ("FPGA API out"=w524:refnum<class "FPGA API.lvclass">, "error out"=w523:errorcluster)  [unwired: 11 in]
            n206 = call-dynamic "Enable Stop Step.vi"("FPGA API in"=w524, "error in (no error)"=w523, "Direction"=Direction."None") -> ("error out"=w518:errorcluster)  [unwired: 11 in, 1 out]
            n207 = call "Close.vi"("Pump_1AI_1DO_2DI in"=w537) -> ("error out"=w531:errorcluster, "Pump_1AI_1DO_2DI out"=w536:refnum<class "Valve_2DO_2DI.lvclass">)  [unwired: 9 in]
            n208 = call "Close.vi"("Pump_1AI_1DO_2DI in"=w535) -> ("error out"=w532:errorcluster, "Pump_1AI_1DO_2DI out"=w534:refnum<class "Valve_2DO_2DI.lvclass">)  [unwired: 9 in]
            n209 = Merge Errors(w518, w531, w532) -> (w533:errorcluster)
          }
          frame "Open Air" {
            w545 = T5 18 items=["DO 0 [KP1] [M12]", "DO 1 [ON KP2] [M21]", "DO 2 [ON KP3] [M24]", "DO 3 [WATER Y18.1 [DO3]]", "DO 4 [WATER Y18.2 [DO4]]", "DO 5 [KP6 Y29.1 33.7]", "DO 6 [KP7 Y29.2 33.8]", "DO 7 [KP8 Y29.3 33.9]", "DO 8 [KP9 Y29.4  33.12]", "DO 9 [KP10 Y29.5 33.1]", "DO 10 [KP11 Y29.6 33.2]", "DO 11 [KP12 Y29.7  33.13]", "DO 12 [KP13 Y29.8  33.11]", "DO 13 [KP14 Y29.9 33.10]", "DO 14 [KP15 Y29.10  33.6]", "DO 15 [KP16 Y29.11  33.5]", "DO 16 [KP17 Y29.12  33.4]", "DO 17 [KP18 Y29.13 33.3]", "DO 18 [AIR KP19]", "DO 19 [STEP DRIVE EN KP20]", "DO 20 [KP21 Y44.1 OPEN]", "DO 21 [ KP22 Y44.1 CLOSE]", "DO 22 [ KP23 Y44.2 OPEN]", "DO 23", "DO 24 [STEP DRIVE 1]", "DO 25 [STEP DRIVE 2]"] ("DO index")
            n210 = call-dynamic "Write Do.vi"("FPGA API in"=w549, "#DO"=w545, "value"=TRUE, "Time uSec"=u32 0, "error in (no error)"=w548) -> ("FPGA API out"=w546:refnum<class "FPGA API.lvclass">, "error out"=w547:errorcluster)  [unwired: 9 in]
            n211 = call-dynamic "SetHasckelAO.vi"("FPGA API in"=w546, "Haskel in"=0.0, "error in (no error)"=w547) -> ("FPGA API out"=w571:refnum<class "FPGA API.lvclass">, "error out"=w570:errorcluster)  [unwired: 11 in]
            n212 = call-dynamic "SetPropValve.vi"("FPGA API in"=w571, "AO 1"=0.0, "error in (no error)"=w570) -> ("FPGA API out"=w563:refnum<class "FPGA API.lvclass">, "error out"=w562:errorcluster)  [unwired: 11 in]
            n213 = call-dynamic "Enable Close Inlet.vi"("FPGA API in"=w563, "error in (no error)"=w562, "Direction"=Direction."None") -> ("FPGA API out"=w560:refnum<class "FPGA API.lvclass">, "error out"=w559:errorcluster)  [unwired: 11 in]
            n214 = call-dynamic "Enable Close Outlet.vi"("FPGA API in"=w560, "error in (no error)"=w559, "Direction"=Direction."None") -> ("FPGA API out"=w557:refnum<class "FPGA API.lvclass">, "error out"=w556:errorcluster)  [unwired: 11 in]
            n215 = call-dynamic "Enable Stop Step.vi"("FPGA API in"=w557, "error in (no error)"=w556, "Direction"=Direction."None") -> ("error out"=w544:errorcluster)  [unwired: 11 in, 1 out]
            n216 = disable-structure shown="Disabled" {
              disable-tunnel: w566 -> [w579 _]
              disable-tunnel: [w577 _] -> w565
              disable-tunnel: w564 -> [w575 _]
              disable-tunnel: [w572 _] -> w554
              frame Disabled {
                # "OPEN"
                # "CLOSE"
                # "STOP"
                n217 = call "GetMessageInterface.vi"("Device in"=w575) -> ("MessageInterface"=w576:refnum<class "MessageInterface.lvclass">)  [unwired: 10 in]
                n218 = call "GetMessageInterface.vi"("Device in"=w579) -> ("MessageInterface"=w578:refnum<class "MessageInterface.lvclass">)  [unwired: 10 in]
                n219 = call-dynamic "SendLocalMsg.vi"("reference in"=w576, "name"="") -> ("error out"=w572:errorcluster)  [unwired: 11 in, 2 out]
                n220 = call-dynamic "SendLocalMsg.vi"("reference in"=w578, "name"="") -> ("error out"=w577:errorcluster)  [unwired: 11 in, 2 out]
              }
              frame Enabled {
              }
            }
            n221 = Merge Errors(w544, w565, w554) -> (w567:errorcluster)
          }
        }
        n222 = in-place-cluster #1("VLV 44.1"=w20, "VLV 44.2"=w19) -> (w12:refnum<class "Stand.lvclass">)
      }
    }
    frame False {
      n223 = in-place {
        in-place-border: [w597] -> w580
        in-place-border: w583 -> [w596]
        in-place-border: w582 -> [w586]
        n224 = in-place-cluster #2(w582) -> ("STEP"=w584:T1, "PM"=w594:refnum<class "PM_Group.lvclass">, "VLV 44.1"=w593:refnum<class "Valve_2DO_2DI.lvclass">, "VLV 44.2"=w592:refnum<class "Valve_2DO_2DI.lvclass">)
        n225 = Unbundle By Name(w586) -> ("NV_DUT"=w588:refnum<class "NeedleValve.lvclass">, "NV_Chamber"=w587:refnum<class "NeedleValve.lvclass">)
        n226 = call "GetFPGA.vi"("Device in"=w586) -> ("FPGA API.lvclass"=w595:refnum<class "FPGA API.lvclass">)  [unwired: 10 in]
        n227 = case shown="\"Stop Pump\"" w584 {
          selector: w584 -> [w598 w609 w641 w674 _ _ _ _ _ _ w732 w753 _ w779 w794 w799 w841 w849 w857]
          tunnel: w596 -> [w602 w605 w637 w677 w691 w696 w701 w705 w719 w724 w735 w756 w770 w782 w795 w802 w844 w852 w860]
          tunnel: [w602 w604 w636 w667 w691 w696 w701 w703 w719 w724 w725 w747 w770 w772 w795 w825 w845 w853 w861] -> w597
          tunnel: w593 -> [w600 w622 w654 w681 w690 w695 w700 w709 w718 w723 w739 w760 w769 w786 w797 w831 w848 w856 w864]
          tunnel: w592 -> [w599 w621 w653 w679 w688 w693 w698 w708 w716 w721 w737 w758 w767 w784 w796 w827 w846 w854 w862]
          tunnel: w595 -> [_ _ _ w678 _ _ _ _ _ _ w736 w757 _ w783 _ w832 _ _ _]
          tunnel: w594 -> [w601 w607 w639 w680 w689 w694 w699 w706 w717 w722 w738 w759 w768 w785 w798 w830 w847 w855 w863]
          tunnel: [w601 w606 w638 w680 w689 w694 w699 w704 w717 w722 w738 w759 w768 w785 w798 w830 w847 w855 w863] -> w591
          tunnel: w586 -> [_ w615 w647 w669 _ _ _ _ _ _ w727 _ _ w774 _ w829 _ _ _]
          tunnel: [w600 w622 w654 w681 w690 w695 w700 w709 w718 w723 w739 w760 w769 w786 w797 w828 w848 w856 w864] -> w590
          tunnel: [w599 w621 w653 w679 w688 w693 w698 w708 w716 w721 w737 w758 w767 w784 w796 w826 w846 w854 w862] -> w589
          tunnel: w588 -> [_ _ _ _ _ _ _ _ _ _ _ _ _ _ _ w822 _ _ _]
          tunnel: w587 -> [_ _ _ _ _ _ _ _ _ _ _ _ _ _ _ w820 _ _ _]
          tunnel: w586 -> [_ w616 w648 _ _ _ _ _ _ _ _ _ _ _ _ w803 w842 w850 w858]
          tunnel: [w598 w608 w640 w670 Step_Name."NONE" ("stepName") Step_Name."NONE" ("stepName") Step_Name."NONE" ("stepName") Step_Name."NONE" ("STEP") Step_Name."NONE" ("stepName") Step_Name."NONE" ("stepName") w728 w749 Step_Name."NONE" ("stepName") w775 w794 w799 w841 w849 w857] -> w585
          frame "NONE" {
          }
          frame "Filling DUT" {
            w618 = T6 0 items=["AI 0 Cooling Station Level", "AI 1 Cooling Station Temp", "AI 2 Oil Supply Level", "AI 3 Oil Supply Temp", "AI 4 ", "AI 5 Pressure Haskel", "AI 6 Pressure DUT", "AI 7 Pressure Chamber", "AI 8 Pressure Air inlet", "AI 9 Pressure Air outlet", "AI 10 Pressure Messure Line"] ("AI index")
            n228 = Unbundle By Name(w615) -> ("Filling Delta Level [%]"=w614:dbl, "BeginFilingLevel"=w613:dbl)
            n229 = Unbundle By Name(w616) -> ("AIs"=w617:refnum<class "AI.lvclass">[])
            n230 = Index Array(array=w617, index=w618) -> (element=w619:refnum<class "AI.lvclass">)
            n231 = call "Get_Values.vi"("reference in"=w619) -> ("Data"=w620:T7)  [unwired: 14 in]
            n232 = Add(x=w614, y=w613) -> (x+y=w611:dbl)
            n233 = Unbundle By Name(w620) -> ("Stat Data.scl mean 1Hz"=w612:dbl)
            n234 = Greater?(x=w612, y=w611) -> (0:w603:bool)
            n235 = Select(t=Step_Name."NONE" ("stepName"), s=w603, f=w609) -> (s? t:f=w608:T1)
            n236 = case shown="True" w603 {
              tunnel: w607 -> [w623 w628]
              tunnel: [w623 w627] -> w606
              tunnel: w605 -> [w624 w626]
              tunnel: [w624 w625] -> w604
              frame False {
              }
              frame True {
                n237 = for {
                  tunnel: T3[] [{"Active"=FALSE, "MotorN"=enum."M12"}, {"Active"=FALSE, "MotorN"=enum."M21"}, {"Active"=FALSE, "MotorN"=enum."M24"}] ("Array") -> [w632] mode=indexing
                  shift-right: [w631] -> w627
                  shift-left: w628 -> [w634]
                  shift-right: [w630] -> w625
                  shift-left: w626 -> [w633]
                  n238 = call "Activate Motor.vi"("reference in"=w634, "Active Motor"=w632, "error in (no error)"=w633) -> ("reference out"=w631:refnum<class "PM_Group.lvclass">, "error out"=w630:errorcluster)  [unwired: 11 in]
                }
              }
            }
          }
          frame "Filling Chamber" {
            w650 = T6 0 items=["AI 0 Cooling Station Level", "AI 1 Cooling Station Temp", "AI 2 Oil Supply Level", "AI 3 Oil Supply Temp", "AI 4 ", "AI 5 Pressure Haskel", "AI 6 Pressure DUT", "AI 7 Pressure Chamber", "AI 8 Pressure Air inlet", "AI 9 Pressure Air outlet", "AI 10 Pressure Messure Line"] ("AI index")
            n239 = Unbundle By Name(w647) -> ("Filling Delta Level [%]"=w646:dbl, "BeginFilingLevel"=w645:dbl)
            n240 = Unbundle By Name(w648) -> ("AIs"=w649:refnum<class "AI.lvclass">[])
            n241 = Index Array(array=w649, index=w650) -> (element=w651:refnum<class "AI.lvclass">)
            n242 = call "Get_Values.vi"("reference in"=w651) -> ("Data"=w652:T7)  [unwired: 14 in]
            n243 = Add(x=w646, y=w645) -> (x+y=w643:dbl)
            n244 = Unbundle By Name(w652) -> ("Stat Data.scl mean 1Hz"=w644:dbl)
            n245 = Greater?(x=w644, y=w643) -> (0:w635:bool)
            n246 = Select(t=Step_Name."NONE" ("stepName"), s=w635, f=w641) -> (s? t:f=w640:T1)
            n247 = case shown="True" w635 {
              tunnel: w639 -> [w655 w660]
              tunnel: [w655 w659] -> w638
              tunnel: w637 -> [w656 w658]
              tunnel: [w656 w657] -> w636
              frame False {
              }
              frame True {
                n248 = for {
                  tunnel: T3[] [{"Active"=FALSE, "MotorN"=enum."M12"}, {"Active"=FALSE, "MotorN"=enum."M21"}, {"Active"=FALSE, "MotorN"=enum."M24"}] ("Array") -> [w664] mode=indexing
                  shift-right: [w663] -> w659
                  shift-left: w660 -> [w666]
                  shift-right: [w662] -> w657
                  shift-left: w658 -> [w665]
                  n249 = call "Activate Motor.vi"("reference in"=w666, "Active Motor"=w664, "error in (no error)"=w665) -> ("reference out"=w663:refnum<class "PM_Group.lvclass">, "error out"=w662:errorcluster)  [unwired: 11 in]
                }
              }
            }
          }
          frame "Pressure Up DUT" {
            w675 = T5 9 items=["DO 0 [KP1] [M12]", "DO 1 [ON KP2] [M21]", "DO 2 [ON KP3] [M24]", "DO 3 [WATER Y18.1 [DO3]]", "DO 4 [WATER Y18.2 [DO4]]", "DO 5 [KP6 Y29.1 33.7]", "DO 6 [KP7 Y29.2 33.8]", "DO 7 [KP8 Y29.3 33.9]", "DO 8 [KP9 Y29.4  33.12]", "DO 9 [KP10 Y29.5 33.1]", "DO 10 [KP11 Y29.6 33.2]", "DO 11 [KP12 Y29.7  33.13]", "DO 12 [KP13 Y29.8  33.11]", "DO 13 [KP14 Y29.9 33.10]", "DO 14 [KP15 Y29.10  33.6]", "DO 15 [KP16 Y29.11  33.5]", "DO 16 [KP17 Y29.12  33.4]", "DO 17 [KP18 Y29.13 33.3]", "DO 18 [AIR KP19]", "DO 19 [STEP DRIVE EN KP20]", "DO 20 [KP21 Y44.1 OPEN]", "DO 21 [ KP22 Y44.1 CLOSE]", "DO 22 [ KP23 Y44.2 OPEN]", "DO 23", "DO 24 [STEP DRIVE 1]", "DO 25 [STEP DRIVE 2]"] ("DO index")
            n250 = call-dynamic "Read DO.vi"("FPGA API in"=w678, "error in (no error)"=w677) -> ("FPGA API out"=w668:refnum<class "FPGA API.lvclass">, "Ds"=w676:bool[], "error out"=w672:errorcluster)  [unwired: 11 in]
            n251 = Index Array(array=w676, index=w675) -> (element=w671:bool)
            n252 = Select(t=Step_Name."NONE", s=w671, f=w674) -> (s? t:f=w670:T1)
            n253 = case shown="True" w671 {
              tunnel: w672 -> [w682 w685]
              tunnel: w669 -> [_ _]
              tunnel: w668 -> [_ w686]
              tunnel: [w682 w683] -> w667
              frame False {
              }
              frame True {
                n254 = call-dynamic "Enable Close Inlet.vi"("FPGA API in"=w686, "error in (no error)"=w685, "Direction"=Direction."None") -> ("error out"=w683:errorcluster)  [unwired: 11 in, 1 out]
              }
            }
          }
          frame "Abrupt Pressure Release DUT" {
          }
          frame "MicroStep DUT" {
          }
          frame "MicroStep CMBR" {
          }
          frame "Stop Pump" {
            n255 = for {
              tunnel: T3[] [{"Active"=FALSE, "MotorN"=enum."M12"}, {"Active"=FALSE, "MotorN"=enum."M21"}, {"Active"=FALSE, "MotorN"=enum."M24"}] ("Array") -> [w712] mode=indexing
              shift-right: [w711] -> w704
              shift-left: w706 -> [w714]
              shift-right: [w710] -> w703
              shift-left: w705 -> [w713]
              n256 = call "Activate Motor.vi"("reference in"=w714, "Active Motor"=w712, "error in (no error)"=w713) -> ("reference out"=w711:refnum<class "PM_Group.lvclass">, "error out"=w710:errorcluster)  [unwired: 11 in]
            }
          }
          frame "ALARM" {
          }
          frame "Open Air" {
          }
          frame "Smooth Pressure Release DUT" {
            w733 = T5 17 items=["DO 0 [KP1] [M12]", "DO 1 [ON KP2] [M21]", "DO 2 [ON KP3] [M24]", "DO 3 [WATER Y18.1 [DO3]]", "DO 4 [WATER Y18.2 [DO4]]", "DO 5 [KP6 Y29.1 33.7]", "DO 6 [KP7 Y29.2 33.8]", "DO 7 [KP8 Y29.3 33.9]", "DO 8 [KP9 Y29.4  33.12]", "DO 9 [KP10 Y29.5 33.1]", "DO 10 [KP11 Y29.6 33.2]", "DO 11 [KP12 Y29.7  33.13]", "DO 12 [KP13 Y29.8  33.11]", "DO 13 [KP14 Y29.9 33.10]", "DO 14 [KP15 Y29.10  33.6]", "DO 15 [KP16 Y29.11  33.5]", "DO 16 [KP17 Y29.12  33.4]", "DO 17 [KP18 Y29.13 33.3]", "DO 18 [AIR KP19]", "DO 19 [STEP DRIVE EN KP20]", "DO 20 [KP21 Y44.1 OPEN]", "DO 21 [ KP22 Y44.1 CLOSE]", "DO 22 [ KP23 Y44.2 OPEN]", "DO 23", "DO 24 [STEP DRIVE 1]", "DO 25 [STEP DRIVE 2]"] ("DO index")
            n257 = call-dynamic "Read DO.vi"("FPGA API in"=w736, "error in (no error)"=w735) -> ("FPGA API out"=w726:refnum<class "FPGA API.lvclass">, "Ds"=w734:bool[], "error out"=w730:errorcluster)  [unwired: 11 in]
            n258 = Index Array(array=w734, index=w733) -> (element=w729:bool)
            n259 = Select(t=Step_Name."NONE", s=w729, f=w732) -> (s? t:f=w728:T1)
            n260 = case shown="True" w729 {
              tunnel: w730 -> [w740 w743]
              tunnel: w727 -> [_ _]
              tunnel: w726 -> [_ w746]
              tunnel: [w740 w741] -> w725
              frame False {
              }
              frame True {
                w744 = Direction."None" ("Direction")
                n261 = call-dynamic "Enable Close Outlet.vi"("FPGA API in"=w746, "error in (no error)"=w743, "Direction"=w744) -> ("FPGA API out"=w745:refnum<class "FPGA API.lvclass">, "error out"=w742:errorcluster)  [unwired: 11 in]
                n262 = call-dynamic "Enable Stop Step.vi"("FPGA API in"=w745, "error in (no error)"=w742, "Direction"=w744) -> ("error out"=w741:errorcluster)  [unwired: 11 in, 1 out]
              }
            }
          }
          frame "Pressure Up Chamber" {
            w754 = T5 10 items=["DO 0 [KP1] [M12]", "DO 1 [ON KP2] [M21]", "DO 2 [ON KP3] [M24]", "DO 3 [WATER Y18.1 [DO3]]", "DO 4 [WATER Y18.2 [DO4]]", "DO 5 [KP6 Y29.1 33.7]", "DO 6 [KP7 Y29.2 33.8]", "DO 7 [KP8 Y29.3 33.9]", "DO 8 [KP9 Y29.4  33.12]", "DO 9 [KP10 Y29.5 33.1]", "DO 10 [KP11 Y29.6 33.2]", "DO 11 [KP12 Y29.7  33.13]", "DO 12 [KP13 Y29.8  33.11]", "DO 13 [KP14 Y29.9 33.10]", "DO 14 [KP15 Y29.10  33.6]", "DO 15 [KP16 Y29.11  33.5]", "DO 16 [KP17 Y29.12  33.4]", "DO 17 [KP18 Y29.13 33.3]", "DO 18 [AIR KP19]", "DO 19 [STEP DRIVE EN KP20]", "DO 20 [KP21 Y44.1 OPEN]", "DO 21 [ KP22 Y44.1 CLOSE]", "DO 22 [ KP23 Y44.2 OPEN]", "DO 23", "DO 24 [STEP DRIVE 1]", "DO 25 [STEP DRIVE 2]"] ("DO index")
            n263 = call-dynamic "Read DO.vi"("FPGA API in"=w757, "error in (no error)"=w756) -> ("FPGA API out"=w748:refnum<class "FPGA API.lvclass">, "Ds"=w755:bool[], "error out"=w751:errorcluster)  [unwired: 11 in]
            n264 = Index Array(array=w755, index=w754) -> (element=w750:bool)
            n265 = Select(t=Step_Name."NONE", s=w750, f=w753) -> (s? t:f=w749:T1)
            n266 = case shown="True" w750 {
              tunnel: w751 -> [w761 w764]
              tunnel: w748 -> [_ w765]
              tunnel: [w761 w762] -> w747
              frame False {
              }
              frame True {
                n267 = call-dynamic "Enable Close Inlet.vi"("FPGA API in"=w765, "error in (no error)"=w764, "Direction"=Direction."None") -> ("error out"=w762:errorcluster)  [unwired: 11 in, 1 out]
              }
            }
          }
          frame "Abrupt Pressure Release Chamber" {
          }
          frame "Smooth Pressure Release Chamber" {
            w771 = T5 24 items=["DO 0 [KP1] [M12]", "DO 1 [ON KP2] [M21]", "DO 2 [ON KP3] [M24]", "DO 3 [WATER Y18.1 [DO3]]", "DO 4 [WATER Y18.2 [DO4]]", "DO 5 [KP6 Y29.1 33.7]", "DO 6 [KP7 Y29.2 33.8]", "DO 7 [KP8 Y29.3 33.9]", "DO 8 [KP9 Y29.4  33.12]", "DO 9 [KP10 Y29.5 33.1]", "DO 10 [KP11 Y29.6 33.2]", "DO 11 [KP12 Y29.7  33.13]", "DO 12 [KP13 Y29.8  33.11]", "DO 13 [KP14 Y29.9 33.10]", "DO 14 [KP15 Y29.10  33.6]", "DO 15 [KP16 Y29.11  33.5]", "DO 16 [KP17 Y29.12  33.4]", "DO 17 [KP18 Y29.13 33.3]", "DO 18 [AIR KP19]", "DO 19 [STEP DRIVE EN KP20]", "DO 20 [KP21 Y44.1 OPEN]", "DO 21 [ KP22 Y44.1 CLOSE]", "DO 22 [ KP23 Y44.2 OPEN]", "DO 23", "DO 24 [STEP DRIVE 1]", "DO 25 [STEP DRIVE 2]"] ("DO index")
            w780 = T5 16 items=["DO 0 [KP1] [M12]", "DO 1 [ON KP2] [M21]", "DO 2 [ON KP3] [M24]", "DO 3 [WATER Y18.1 [DO3]]", "DO 4 [WATER Y18.2 [DO4]]", "DO 5 [KP6 Y29.1 33.7]", "DO 6 [KP7 Y29.2 33.8]", "DO 7 [KP8 Y29.3 33.9]", "DO 8 [KP9 Y29.4  33.12]", "DO 9 [KP10 Y29.5 33.1]", "DO 10 [KP11 Y29.6 33.2]", "DO 11 [KP12 Y29.7  33.13]", "DO 12 [KP13 Y29.8  33.11]", "DO 13 [KP14 Y29.9 33.10]", "DO 14 [KP15 Y29.10  33.6]", "DO 15 [KP16 Y29.11  33.5]", "DO 16 [KP17 Y29.12  33.4]", "DO 17 [KP18 Y29.13 33.3]", "DO 18 [AIR KP19]", "DO 19 [STEP DRIVE EN KP20]", "DO 20 [KP21 Y44.1 OPEN]", "DO 21 [ KP22 Y44.1 CLOSE]", "DO 22 [ KP23 Y44.2 OPEN]", "DO 23", "DO 24 [STEP DRIVE 1]", "DO 25 [STEP DRIVE 2]"] ("DO index")
            n268 = call-dynamic "Read DO.vi"("FPGA API in"=w783, "error in (no error)"=w782) -> ("FPGA API out"=w773:refnum<class "FPGA API.lvclass">, "Ds"=w781:bool[], "error out"=w777:errorcluster)  [unwired: 11 in]
            n269 = Index Array(array=w781, index #1=w780, index #2=w771) -> (element #1=w776:bool)  [unwired: 1 out]
            n270 = Select(t=Step_Name."NONE", s=w776, f=w779) -> (s? t:f=w775:T1)
            n271 = case shown="True" w776 {
              tunnel: w777 -> [w787 w790]
              tunnel: w774 -> [_ _]
              tunnel: w773 -> [_ w793]
              tunnel: [w787 w788] -> w772
              frame False {
              }
              frame True {
                w791 = Direction."None" ("Direction")
                n272 = call-dynamic "Enable Close Outlet.vi"("FPGA API in"=w793, "error in (no error)"=w790, "Direction"=w791) -> ("FPGA API out"=w792:refnum<class "FPGA API.lvclass">, "error out"=w789:errorcluster)  [unwired: 11 in]
                n273 = call-dynamic "Enable Stop Step.vi"("FPGA API in"=w792, "error in (no error)"=w789, "Direction"=w791) -> ("error out"=w788:errorcluster)  [unwired: 11 in, 1 out]
              }
            }
          }
          frame "Measuring leakage sensor 41.3" {
          }
          frame "Measuring leakage burette 42" {
            w800 = T5[] [8, 17, 10] items=["DO 0 [KP1] [M12]", "DO 1 [ON KP2] [M21]", "DO 2 [ON KP3] [M24]", "DO 3 [WATER Y18.1 [DO3]]", "DO 4 [WATER Y18.2 [DO4]]", "DO 5 [KP6 Y29.1 33.7]", "DO 6 [KP7 Y29.2 33.8]", "DO 7 [KP8 Y29.3 33.9]", "DO 8 [KP9 Y29.4  33.12]", "DO 9 [KP10 Y29.5 33.1]", "DO 10 [KP11 Y29.6 33.2]", "DO 11 [KP12 Y29.7  33.13]", "DO 12 [KP13 Y29.8  33.11]", "DO 13 [KP14 Y29.9 33.10]", "DO 14 [KP15 Y29.10  33.6]", "DO 15 [KP16 Y29.11  33.5]", "DO 16 [KP17 Y29.12  33.4]", "DO 17 [KP18 Y29.13 33.3]", "DO 18 [AIR KP19]", "DO 19 [STEP DRIVE EN KP20]", "DO 20 [KP21 Y44.1 OPEN]", "DO 21 [ KP22 Y44.1 CLOSE]", "DO 22 [ KP23 Y44.2 OPEN]", "DO 23", "DO 24 [STEP DRIVE 1]", "DO 25 [STEP DRIVE 2]"] ("#DO")
            # "Замер утечек из образца по датчику 41.3\n4.1\tконтроль показаний\n4.2\tконтроль показаний\n5.1\tконтроль показаний\n5.2\tконтроль показаний\n12\t0/1\n18.1\t0/1\n18.2\t0/1\n21\t1\n24\t0/1\n25\t1\n29.1 (33.7)\t0\n29.2 (33.8)\t0\n29.3 (33.9)\t0\n29.4 (33.12)\t1\n29.5 (33.1)\t0\n29.6 (33.2)\t1\n29.7 (33.13)\t0\n29.8 (33.11)\t0\n29.9 (33.10)\t0\n29.10 (33.6)\t0\n29.11 (33.5)\t0\n29.12 (33.4)\t0\n29.13 (33.3) \t1\n30\t0…10 В\n35.1\t60%\n35.2\t0\n36.1\tконтроль показаний\n36.2\tконтроль показаний\n38.1\tконтроль показаний\n38.2\tконтроль показаний\n38.3\tобратная связь\n41.3\tконтроль показаний\n44.1\t0\n44.2\t0\n46\t0…1,5 В"
            # "OPEN"
            # "CLOSE"
            # "STOP"
            n274 = Unbundle By Name(w829) -> ("Pressure SP"=w807:dbl)
            n275 = call "Config Setpoints.vi"("reference in"=w803, "error in (no error)"=w802) -> ("error out"=w801:errorcluster)  [unwired: 13 in]
            n276 = call "Pressure to voltage.vi"("Pressure SP"=w807) -> ()  [unwired: 14 in, 1 out]
            n277 = call "Set Valve State.vi"("reference in"=w832, "#DO"=w800, "error in (no error)"=w801) -> ("reference out"=w836:refnum<class "FPGA API.lvclass">, "error out"=w835:errorcluster)  [unwired: 11 in]
            n278 = call-dynamic "SetHasckelAO.vi"("FPGA API in"=w836, "Haskel in"=0.0, "error in (no error)"=w835) -> ("FPGA API out"=w834:refnum<class "FPGA API.lvclass">, "error out"=w833:errorcluster)  [unwired: 11 in]
            n279 = call-dynamic "SetPropValve.vi"("FPGA API in"=w834, "AO 1"=0.0, "error in (no error)"=w833) -> ("FPGA API out"=w819:refnum<class "FPGA API.lvclass">, "error out"=w818:errorcluster)  [unwired: 11 in]
            n280 = call-dynamic "Enable Close Inlet.vi"("FPGA API in"=w819, "error in (no error)"=w818, "Direction"=Direction."None") -> ("FPGA API out"=w816:refnum<class "FPGA API.lvclass">, "error out"=w815:errorcluster)  [unwired: 11 in]
            n281 = call-dynamic "Enable Close Outlet.vi"("FPGA API in"=w816, "error in (no error)"=w815, "Direction"=Direction."Chamber") -> ("FPGA API out"=w813:refnum<class "FPGA API.lvclass">, "error out"=w812:errorcluster)  [unwired: 11 in]
            n282 = call-dynamic "Enable Stop Step.vi"("FPGA API in"=w813, "error in (no error)"=w812, "Direction"=Direction."Chamber") -> ("error out"=w811:errorcluster)  [unwired: 11 in, 1 out]
            n283 = disable-structure shown="Disabled" {
              disable-tunnel: w822 -> [w840 _]
              disable-tunnel: [w839 _] -> w821
              frame Disabled {
                n284 = call "GetMessageInterface.vi"("Device in"=w840) -> ("MessageInterface"=w838:refnum<class "MessageInterface.lvclass">)  [unwired: 10 in]
                n285 = call-dynamic "SendLocalMsg.vi"("reference in"=w838, "name"="") -> ("error out"=w839:errorcluster)  [unwired: 11 in, 2 out]
              }
              frame Enabled {
              }
            }
            n286 = call "GetMessageInterface.vi"("Device in"=w820) -> ("MessageInterface"=w805:refnum<class "MessageInterface.lvclass">)  [unwired: 10 in]
            n287 = call "Close.vi"("Pump_1AI_1DO_2DI in"=w831) -> ("error out"=w823:errorcluster, "Pump_1AI_1DO_2DI out"=w828:refnum<class "Valve_2DO_2DI.lvclass">)  [unwired: 9 in]
            n288 = call "Close.vi"("Pump_1AI_1DO_2DI in"=w827) -> ("error out"=w824:errorcluster, "Pump_1AI_1DO_2DI out"=w826:refnum<class "Valve_2DO_2DI.lvclass">)  [unwired: 9 in]
            n289 = call-dynamic "SendLocalMsg.vi"("reference in"=w805, "name"="OPEN") -> ("error out"=w809:errorcluster)  [unwired: 11 in, 2 out]
            n290 = Merge Errors(w811, w823, w824, w821, w809) -> (w825:errorcluster)
          }
          frame "Low Pressure DUT" {
            w843 = T6 6 items=["AI 0 Cooling Station Level", "AI 1 Cooling Station Temp", "AI 2 Oil Supply Level", "AI 3 Oil Supply Temp", "AI 4 ", "AI 5 Pressure Haskel", "AI 6 Pressure DUT", "AI 7 Pressure Chamber", "AI 8 Pressure Air inlet", "AI 9 Pressure Air outlet", "AI 10 Pressure Messure Line"] ("AI index")
            n291 = call "Set Low Press.vi"("reference in"=w842, "AI index"=w843, "error in (no error)"=w844) -> ("error out"=w845:errorcluster)  [unwired: 12 in]
          }
          frame "Low Pressure Chamber" {
            w851 = T6 7 items=["AI 0 Cooling Station Level", "AI 1 Cooling Station Temp", "AI 2 Oil Supply Level", "AI 3 Oil Supply Temp", "AI 4 ", "AI 5 Pressure Haskel", "AI 6 Pressure DUT", "AI 7 Pressure Chamber", "AI 8 Pressure Air inlet", "AI 9 Pressure Air outlet", "AI 10 Pressure Messure Line"] ("AI index")
            n292 = call "Set Low Press.vi"("reference in"=w850, "AI index"=w851, "error in (no error)"=w852) -> ("error out"=w853:errorcluster)  [unwired: 12 in]
          }
          frame "Low Pressure HPP" {
            w859 = T6 5 items=["AI 0 Cooling Station Level", "AI 1 Cooling Station Temp", "AI 2 Oil Supply Level", "AI 3 Oil Supply Temp", "AI 4 ", "AI 5 Pressure Haskel", "AI 6 Pressure DUT", "AI 7 Pressure Chamber", "AI 8 Pressure Air inlet", "AI 9 Pressure Air outlet", "AI 10 Pressure Messure Line"] ("AI index")
            n293 = call "Set Low Press.vi"("reference in"=w858, "AI index"=w859, "error in (no error)"=w860) -> ("error out"=w861:errorcluster)  [unwired: 12 in]
          }
        }
        n294 = in-place-cluster #2("STEP"=w585, "PM"=w591, "VLV 44.1"=w590, "VLV 44.2"=w589) -> (w581:refnum<class "Stand.lvclass">)
      }
    }
  }
  "error out" <- w7
  "Stand out" <- w8
